vi "MC_10_19a_JW5.vi"() -> ()   [LabVIEW 2011]
uses:
  <vilib>/Utility/file.llb/Read From Spreadsheet File (string).vi
  <vilib>/Utility/inputDevices.llb/keyboardAcquire.vi
  <vilib>/Utility/file.llb/Write To Spreadsheet File (DBL).vi
  <vilib>/Utility/file.llb/Write To Spreadsheet File (string).vi
  <vilib>/regexp/Match Regular Expression.xnode
panel:
  out "Current \nRecord":string[](array[string])
  out "Transformer \nHeaders":string[](array[string])
  out "Current Device ID":string
  out "Column":string
  out "Row":string
  out "Date Recorded":string="Date Recorded"
  out "Concentration Recorded":string
  out "Solvent Recorded":string
  out "Method Recorded":string
  in  "?":T1(tab)
  out "Material Recorded":string
  in  "Treatment Concentration (mM):":dbl=30.0
  in  "Surface Treatment:":string
  in  "# Drops:":dbl=inf
  in  "Solution Temp (C):":dbl=55.0
  in  "Relative Humidity (%):":dbl=nan
  in  "Room Temp (F):":dbl=nan
  in  "Time (s):":dbl=80.0
  out "Accel (RPM/s):":dbl
  in  "RPM:":dbl=1000.0
  in  "Wait Time (s):":dbl=10.0
  in  "Sample #:":dbl=1.0
  in  "Fabricator:":string="Jeremy"
  in  "Data File":path
  out "Data Folder":path
  in  "Image Folder":path
  out "Image File":path
  in  "Ramp (s):":dbl=3.0
  out "Mobility":dbl format="%#_4e"
  out "Length":dbl
  out "Width":dbl
  out "Dielectric (d)":dbl
  out "XY Graph":cluster{dbl[], dbl[]}[](graph)
  in  "NumPts":dbl=5.0
  in  "Cancel Button":bool
  in  "Next Button":bool
  in  "Previous Button":bool
  in  "Up Button":bool
  in  "Down Button":bool
  out "Data Name":string
  in  "Save Changes?":bool
  in  "New Dielectric":dbl
  in  "New Length":dbl
  in  "New Width":dbl
  out "New Mobility":dbl format="%#_4e"
  in  "Slide":dbl(slide) step=1.0 scale=-14.3..84.0 scale format="%#_1p"
  in  "Blank Button":bool
  in  "Zoom":i16(slide)=-3 scale=-5.0..5.0
  out "Image Out 2":T2(plugin-control)
  out "Image Out":T2(plugin-control)
  in  "Magnification":u16(ring) items=["5x", "10x", "20x", "50x", "80x"]
  out "Total Width":dbl
  out "Distances":dbl[](array[numeric])
  in  "Undo Button":bool
  in  "Remove Button":bool
  out "Recorded Mobility":dbl format="%#_4e"
  out "Index 3":string
  out "Image Name":string
  in  "Export":bool
  out "Threshold V":dbl
  out "New Vt":dbl
  in  "Manual":bool
  out "XY Graph 2":cluster{dbl[], dbl[]}[](graph)
  in  "Next Button 2":bool
  in  "Previous Button 2":bool
  in  "Slide 2":dbl(slide) step=1.0 scale=-1.0..82.0 scale format="%#_1p"
  out "S.T.S.":dbl
  out "New S.T.S.":dbl
  in  "NumPts 2":dbl=5.0
  out "Vt recorded":dbl
  out "STS recorded":dbl
  out "On/Off":dbl format="%#_3e"
  in  "Save Changes? 2":bool
  in  "Save Changes? 3":bool
  out "String":string
  in  "No Image":path=path "C:/Program Files/Mega Awesome/Image Not Found.png"
  in  "Project":path=path "C:/Program Files/Mega Awesome/DeviceData.opj"
  out "Index 2":dbl
  out "Array 8":dbl[](array[numeric])
  out "Array 7":dbl[](array[numeric])
  out "ROI Descriptor out":T3 {"Contours"."Type" items=["No Selection", "Point", "Line", "Rectangle", "Oval", "Polygon", "Freehand Region", "Annulus", "Unused2", "Unused3", "Broken Line", "Freehand Line", "Rotated Rectangle"]}
  out "ROI Descriptor":T3 {"Contours"."Type" items=["No Selection", "Point", "Line", "Rectangle", "Oval", "Polygon", "Freehand Region", "Annulus", "Unused2", "Unused3", "Broken Line", "Freehand Line", "Rotated Rectangle"]}
  out "Numeric 3":dbl
  out "Array 6":dbl[][](array[numeric])
  out "Cluster":T4
  out "Array 5":dbl[](array[numeric])
  out "Array 4":dbl[](array[numeric])
  out "Array 3":dbl[](array[numeric])
  out "Numeric 2":dbl
  out "Numeric":dbl
  out "Array 2":dbl[](array[numeric])
  out "Array":dbl[](array[numeric])
  out "Index":dbl
  out "Table Control 2":string[][](table)
  out "Table Control":string[][](table)
  in  "Row Start":dbl=20.0
  # "Data Locations"
  # "Data Location"
  # "Image Location"
  # "Sample Properties"
  # "Recorded"
  # "Calculated"
  # "Re-Calculated"
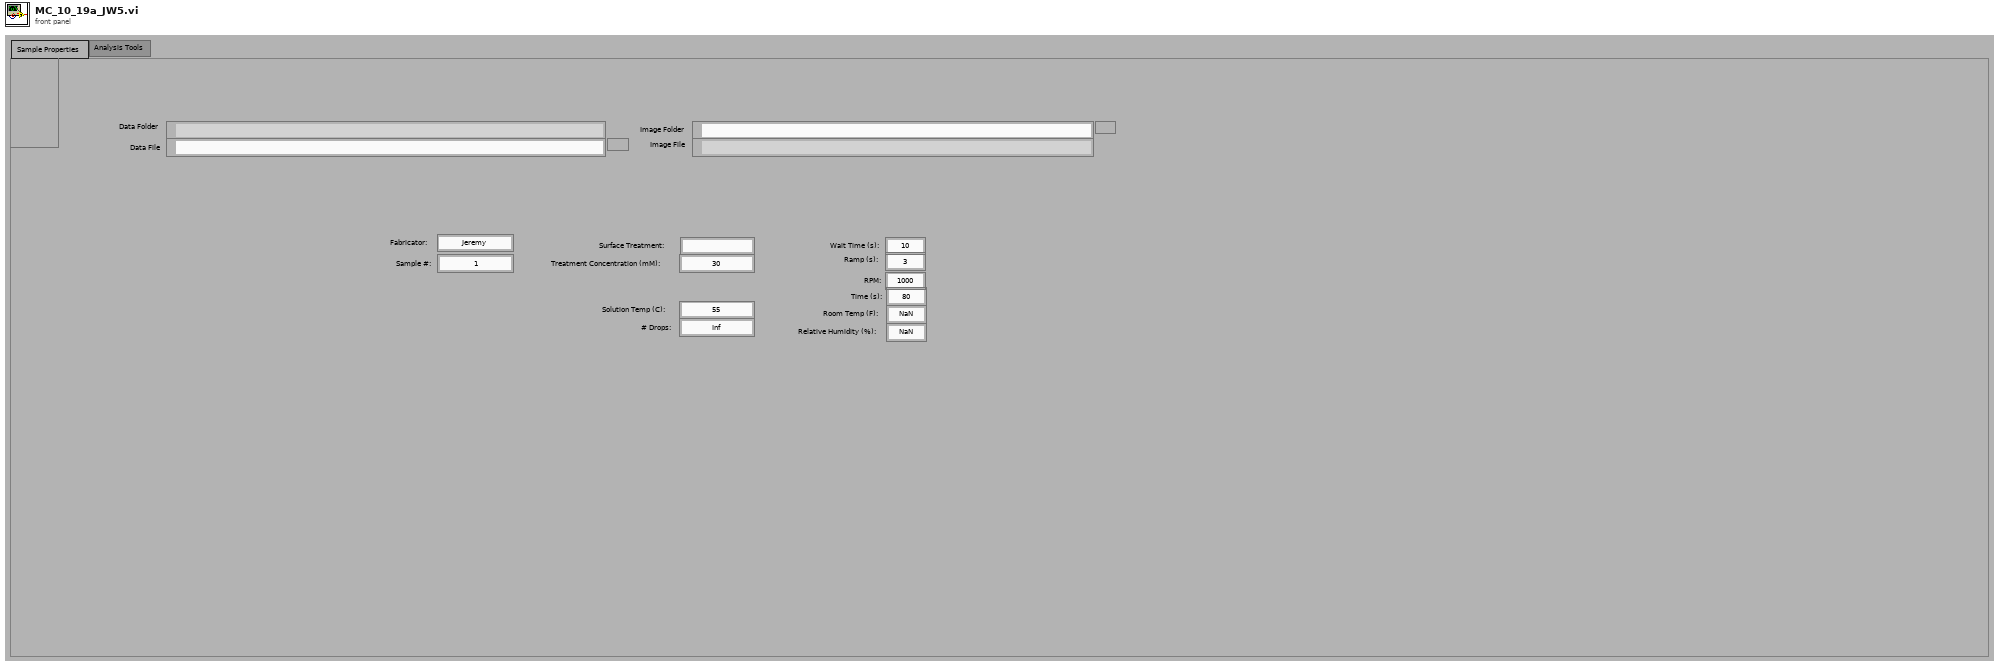
[diagram p1: front panel]
types:
  T1 = enum32{"Sample Properties", "Analysis Tools", "Current Database"}
  T2 = typedef "IMAQ Image.ctl" = refnum<image>
  T3 = typedef "ROI Descriptor" = cluster{"Global Rectangle":i32[], "Contours":cluster{"ID":enum32{"External", "Internal"}, "Type":u32, "Coordinates":i32[]}[]}
  T4 = cluster{"Numeric":dbl, "Numeric 2":dbl, "Numeric 3":dbl, "Numeric 4":dbl}
  T5 = cluster{"[0]":cluster{dbl[], dbl[]}, "[1]":cluster{dbl[], dbl[]}, "[2]":cluster{dbl[], dbl[]}, "[3]":cluster{dbl[], dbl[]}, "[4]":cluster{dbl[], dbl[]}, "[5]":cluster{dbl[], dbl[]}, "[6]":cluster{dbl[], dbl[]}, "[7]":cluster{dbl[], dbl[]}, "[8]":cluster{dbl[], dbl[]}}
  T6 = cluster{"Vt":dbl, "STS":dbl, "On/Off":dbl, "Deposition":string, "Solvent":string, "Concentration":string, "Material":string}
  T7 = cluster{"Global Rectangle":i32[], "Contours":cluster{"Contour Type":u32, "ROI Type":u32, "Points":i32[]}[]}
  T8 = typedef "LVBoundsTypeDef.ctl" = cluster{"Width":u32, "Height":u32}
  T9 = cluster{"Contour Type":u32, "ROI Type":u32, "Points":i32[]}[]
  T10 = enum16{"0", "1", "2", "3", "4", "5", "6", "7", "8", "9", "A", "B", "C", "D", "E", "F", "G", "H", "I", "J", "K", "L", "M", "N", "O", "P", "Q", "R", "S", "T", "U", "V", "W", "X", "Y", "Z", "F1", "F2", "F3", "F4", "F5", "F6", "F7", "F8", "F9", "F10", "F11", "F12", "F13", "F14", "F15", "ADD", "BACK", "BACKSLASH", "CAPITAL", "COMMA", "DECIMAL", "DELETE", "DIVIDE", "DOWN", "END", "EQUALS", "ESCAPE", "GRAVE (`)", "HOME", "INSERT", "LBRACKET", "LCONTROL", "LEFT", "L ALT", "LSHIFT", "LWIN", "MINUS", "MULTIPLY", "NEXT", "NUMLOCK", "NUMPAD_0", "NUMPAD_1", "NUMPAD_2", "NUMPAD_3", "NUMPAD_4", "NUMPAD_5", "NUMPAD_6", "NUMPAD_7", "NUMPAD_8", "NUMPAD_9", "PAUSE", "PERIOD", "PRIOR (PG UP)", "RBRACKET", "RCONTROL", "RETURN", "RIGHT", "R ALT", "RSHIFT", "RWIN", "SCROLL", "SEMICOLON", "SLASH", "SPACE", "SUBTRACT", "TAB", "UP", "ENTER (num pad)", "' (quote)"}[]
  T11 = cluster{i32[], cluster{"Contour Type":u32, "ROI Type":u32, "Points":i32[]}[]}
  T12 = enum16{"0", "1", "2", "3", "4", "5", "6", "7", "8", "9", "A", "B", "C", "D", "E", "F", "G", "H", "I", "J", "K", "L", "M", "N", "O", "P", "Q", "R", "S", "T", "U", "V", "W", "X", "Y", "Z", "F1", "F2", "F3", "F4", "F5", "F6", "F7", "F8", "F9", "F10", "F11", "F12", "F13", "F14", "F15", "ADD", "BACK", "BACKSLASH", "CAPITAL", "COMMA", "DECIMAL", "DELETE", "DIVIDE", "DOWN", "END", "EQUALS", "ESCAPE", "GRAVE (`)", "HOME", "INSERT", "LBRACKET", "LCONTROL", "LEFT", "L ALT", "LSHIFT", "LWIN", "MINUS", "MULTIPLY", "NEXT", "NUMLOCK", "NUMPAD_0", "NUMPAD_1", "NUMPAD_2", "NUMPAD_3", "NUMPAD_4", "NUMPAD_5", "NUMPAD_6", "NUMPAD_7", "NUMPAD_8", "NUMPAD_9", "PAUSE", "PERIOD", "PRIOR (PG UP)", "RBRACKET", "RCONTROL", "RETURN", "RIGHT", "R ALT", "RSHIFT", "RWIN", "SCROLL", "SEMICOLON", "SLASH", "SPACE", "SUBTRACT", "TAB", "UP", "ENTER (num pad)", "' (quote)"}
  T13 = cluster{string, sgl, bool, bool, bool, bool, bool, bool, i32}
  T14 = cluster{i32, cluster{string, sgl, bool, bool, bool, bool, bool, bool, i32}, i32, i32}
  T15 = cluster{"Contour Type":u32, "ROI Type":u32, "Points":i32[]}
  T16 = cluster{"Points[0]":i32, "Points[1]":i32, "Points[2]":i32, "Points[3]":i32, "Points[4]":i32, "Points[5]":i32, "Points[6]":i32, "Points[7]":i32, "Points[8]":i32}
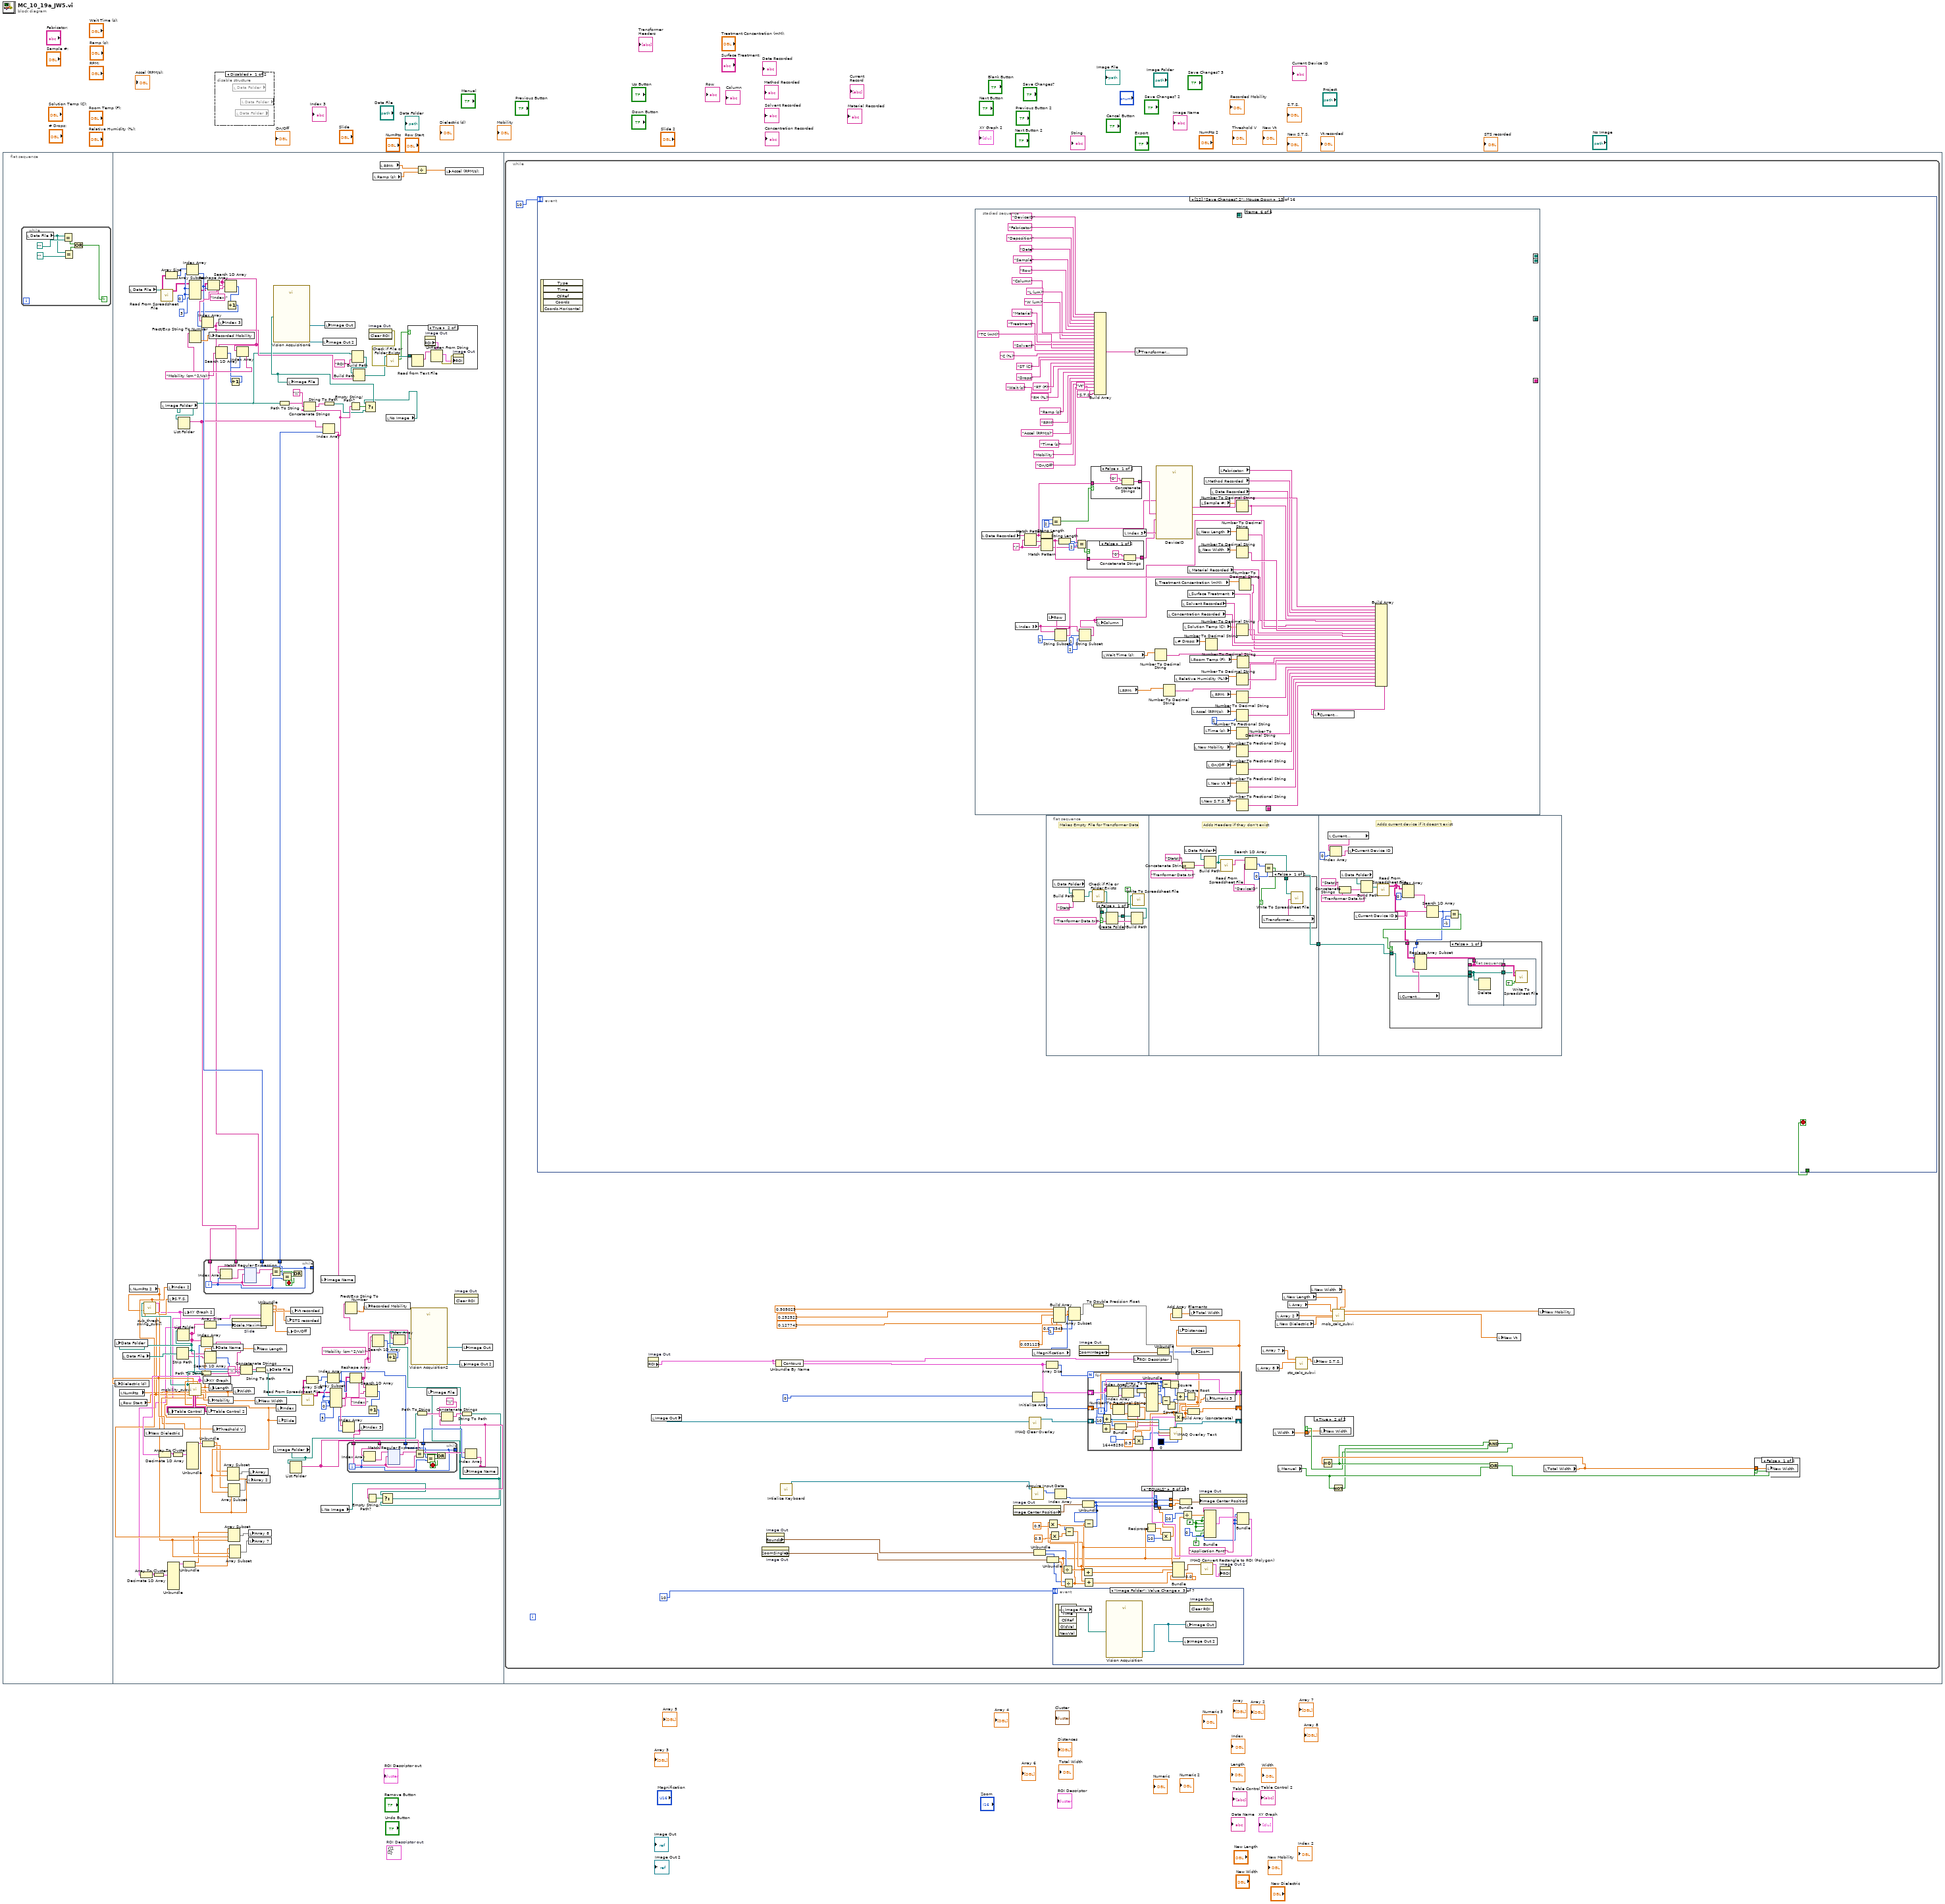
[diagram p0: block diagram]
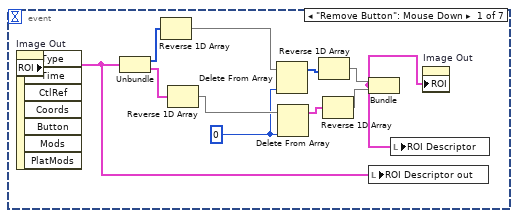
[diagram p5: hidden frame]
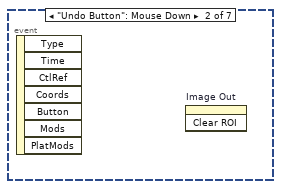
[diagram p6: hidden frame]
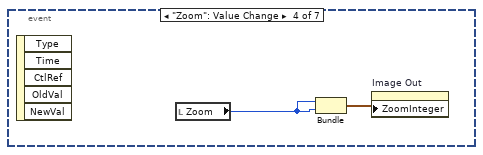
[diagram p7: hidden frame]
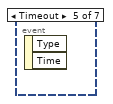
[diagram p8: hidden frame]
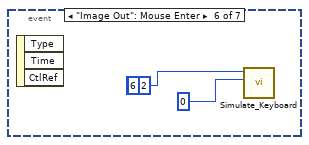
[diagram p9: hidden frame]
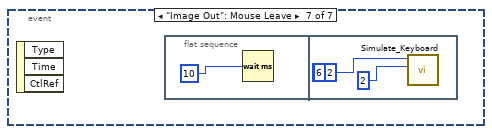
[diagram p10: hidden frame]
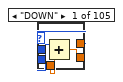
[diagram p11: hidden frame]
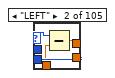
[diagram p12: hidden frame]
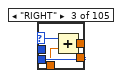
[diagram p13: hidden frame]
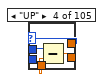
[diagram p14: hidden frame]
diagram:
  (unwired) T3 {"Global Rectangle"=[], "Contours"=[]}  # ROI Descriptor out
  n1 = flat-sequence {
    frame #0 {
      n2 = while {
        stop <- w1 continue-if-true
        n3 = local read "Data File"() -> (w3:path)
        n4 = Equal?(x=w3, y=path "") -> (x = y?=w5:bool)
        n5 = Equal?(x=w3, y=path "") -> (x = y?=w4:bool)
        n6 = Or(x=w5, y=w4) -> (x .or. y?=w1:bool)
      }
    }
    frame #1 {
      w70 = 0
      w100 = 0
      n7 = local read "NumPts"() -> (w45:dbl)
      n8 = local read "Row Start"() -> (w44:dbl)
      n9 = local read "Data File"() -> (w74:path)
      n10 = local read "Data File"() -> (w95:path)
      n11 = local read "NumPts 2"() -> (w39:dbl)
      n12 = call-poly <vilib>:"Read From Spreadsheet File.vi"("file path (dialog if empty)"=w95) -> ("all rows"=w98:string[][])  [unwired: 6 in, 4 out]
      n13 = local read "Image Folder"() -> (w10:path)
      n14 = Array Size(array=w98) -> (size(s)=w99:i32[])
      n15 = Strip Path(path=w74) -> (stripped path=w75:path, name=w56:string)
      n16 = local write "Data Folder"(w75) -> ()
      n17 = List Folder(path=w75) -> (filenames=w64:string[])  [unwired: 3 in, 3 out]
      n18 = List Folder(path=w10) -> (filenames=w104:string[])  [unwired: 3 in, 3 out]
      n19 = Index Array(array=w99, index=w100) -> (element=w106:i32)
      n20 = Array Subset(array=w98, index (row)=w100, index (col)=w100, length (col)=3) -> (w97:string[][])  [unwired: 1 in]
      n21 = Path To String(path=w75) -> (string=w55:string)
      n22 = Array Size(array=w64) -> (size(s)=w65:i32)
      n23 = Search 1D Array(1D array=w64, element=w56) -> (index of element=w63:i32)  [unwired: 1 in]
      n24 = Index Array(array=w64, index=w63) -> (element=w62:string)
      n25 = Reshape Array(w97, w106) -> (w116:string[])
      n26 = local write "Data Name"(w62) -> ()
      n27 = Search 1D Array(1D array=w116, element="Mobility (cm^2/Vs):") -> (index of element=w111:i32)  [unwired: 1 in]
      n28 = Search 1D Array(1D array=w116, element="Index:") -> (index of element=w103:i32)  [unwired: 1 in]
      n29 = Increment(x=w103) -> (x+1=w102:i32)
      n30 = Index Array(array=w116, index=w102) -> (element=w11:string)
      n31 = while {
        tunnel: w104 -> [w249]
        tunnel: w11 -> [w247]
        tunnel: [w246] -> _
        tunnel: [w246] -> w105
        tunnel: w106 -> [w245]
        i -> [w246]
        stop <- w242 stop-if-true
        n32 = Index Array(array=w249, index=w246) -> (element=w250:string)
        n33 = xnode "Match Regular Expression"("input string"=w250, "regular expression"=w247) -> ("whole match"=w248:string)  [unwired: 4 in, 4 out]
        n34 = Equal?(x=w248, y=w247) -> (x = y?=w244:bool)
        n35 = Equal?(x=w245, y=w246) -> (x = y?=w243:bool)
        n36 = Or(x=w244, y=w243) -> (x .or. y?=w242:bool)
      }
      n37 = local write "Index 3"(w11) -> ()
      n38 = Increment(x=w111) -> (x+1=w112:i32)
      n39 = property on="Slide" class="Slide (strict)"("Scale.Maximum"=w65) -> ()  [unwired: 2 in, 2 out]
      n40 = Index Array(array=w116, index=w112) -> (element=w114:string)
      n41 = Fract/Exp String To Number(string=w114) -> (number=w115:dbl)  [unwired: 3 in, 1 out]
      n42 = local write "Recorded Mobility"(w115) -> ()
      n43 = Concatenate Strings(w55, "\\", w62) -> (w57:string)
      n44 = String To Path(string=w57) -> (path=w46:path)
      n45 = call "sub_thresh_swing_subvi.vi"("Path"=w46, "NumPts"=w39, "Row Start"=w44) -> ("Index"=w40:dbl, "XY Graph"=w35:cluster{dbl[], dbl[]}[], "Sub Threshold Swing"=w47:dbl)  [unwired: 8 in, 2 out]
      n46 = Decimate 1D Array(w35) -> (w36:cluster{dbl[], dbl[]}[])  [unwired: 1 out]
      n47 = Array To Cluster(array=w36) -> (cluster=w38:T5)
      n48 = local write "Index 2"(w40) -> ()
      n49 = Unbundle(w38) -> ("[0]"=w37:cluster{dbl[], dbl[]})  [unwired: 8 out]
      n50 = local write "S.T.S."(w47) -> ()
      n51 = local write "XY Graph 2"(w35) -> ()
      n52 = Unbundle(w37) -> (w33:dbl[], w32:dbl[])
      n53 = call "mobility_subvi.vi"("Path"=w46, "NumPts"=w45, "Row Start"=w44) -> ("Dielectric (d)"=w51:dbl, "Index"=w52:dbl, "XY Graph"=w94:cluster{dbl[], dbl[]}[], "Length"=w50:dbl, "Vt"=w48:dbl, "Width"=w49:dbl, "Table Control"=w59:string[][], "Table Control 2"=w60:string[][], "Recorded"=w29:T6, "Mobility"=w61:dbl)  [unwired: 2 in, 1 out]
      n54 = local write "Dielectric (d)"(w51) -> ()
      n55 = local write "New Dielectric"(w51) -> ()
      n56 = Decimate 1D Array(w94) -> (w93:cluster{dbl[], dbl[]}[])  [unwired: 1 out]
      n57 = local write "Table Control"(w59) -> ()
      n58 = Array To Cluster(array=w93) -> (cluster=w91:T5)
      n59 = Unbundle(w91) -> ("[0]"=w92:cluster{dbl[], dbl[]})  [unwired: 8 out]
      n60 = Unbundle(w92) -> (w34:dbl[], w41:dbl[])
      n61 = local write "XY Graph"(w94) -> ()
      n62 = local write "Table Control 2"(w60) -> ()
      n63 = local write "Mobility"(w61) -> ()
      n64 = local write "Length"(w50) -> ()
      n65 = local write "Threshold V"(w48) -> ()
      n66 = Array Subset(array=w34, index=w52, length=w45) -> (w53:dbl[])
      n67 = Array Subset(array=w41, index=w52, length=w45) -> (w54:dbl[])
      n68 = Array Subset(array=w33, index=w40, length=w39) -> (w43:dbl[])
      n69 = Array Subset(array=w32, index=w40, length=w39) -> (w42:dbl[])
      n70 = local write "Width"(w49) -> ()
      n71 = local write "Array 2"(w54) -> ()
      n72 = local write "Array 8"(w43) -> ()
      n73 = local write "Array 7"(w42) -> ()
      n74 = local write "Array"(w53) -> ()
      n75 = local write "New Length"(w50) -> ()
      n76 = local write "New Width"(w49) -> ()
      n77 = Unbundle(w29) -> ("Vt"=w31:dbl, "STS"=w30:dbl, "On/Off"=w28:dbl)  [unwired: 4 out]
      n78 = local write "Data File"(w46) -> ()
      n79 = local read "Image Folder"() -> (w81:path)
      n80 = local write "Index"(w52) -> ()
      n81 = local write "Slide"(w52) -> ()
      n82 = Path To String(path=w10) -> (string=w108:string)
      n83 = local write "STS recorded"(w30) -> ()
      n84 = local write "On/Off"(w28) -> ()
      n85 = List Folder(path=w81) -> (filenames=w77:string[])  [unwired: 3 in, 3 out]
      n86 = local write "Vt recorded"(w31) -> ()
      n87 = call-poly <vilib>:"Read From Spreadsheet File.vi"("file path (dialog if empty)"=w46) -> ("all rows"=w68:string[][])  [unwired: 6 in, 4 out]
      n88 = Array Size(array=w68) -> (size(s)=w69:i32[])
      n89 = local read "No Image"() -> (w19:path)
      n90 = Index Array(array=w104, index=w105) -> (element=w27:string)
      n91 = Concatenate Strings(w108, "\\", w27) -> (w109:string)
      n92 = local write "Image Name"(w27) -> ()
      n93 = String To Path(string=w109) -> (path=w25:path)
      n94 = Index Array(array=w69, index=w70) -> (element=w80:i32)
      n95 = Array Subset(array=w68, index (row)=w70, index (col)=w70, length (col)=3) -> (w67:string[][])  [unwired: 1 in]
      n96 = Empty String/Path?(string/path=w27) -> (empty?=w26:bool)
      n97 = Reshape Array(w67, w80) -> (w90:string[])
      n98 = Build Path(base path=w10, name or relative path="ROI") -> (appended path=w13:path)
      n99 = Build Path(base path=w13, name or relative path=w11) -> (appended path=w12:path)
      n100 = Search 1D Array(1D array=w90, element="Index:") -> (index of element=w73:i32)  [unwired: 1 in]
      n101 = Increment(x=w73) -> (x+1=w72:i32)
      n102 = Index Array(array=w90, index=w72) -> (element=w78:string)
      n103 = while {
        tunnel: w77 -> [w129]
        tunnel: w78 -> [w127]
        tunnel: [w126] -> _
        tunnel: [w126] -> w79
        tunnel: w80 -> [w125]
        i -> [w126]
        stop <- w122 stop-if-true
        n104 = Index Array(array=w129, index=w126) -> (element=w130:string)
        n105 = xnode "Match Regular Expression"("input string"=w130, "regular expression"=w127) -> ("whole match"=w128:string)  [unwired: 4 in, 4 out]
        n106 = Equal?(x=w128, y=w127) -> (x = y?=w124:bool)
        n107 = Equal?(x=w125, y=w126) -> (x = y?=w123:bool)
        n108 = Or(x=w124, y=w123) -> (x .or. y?=w122:bool)
      }
      n109 = local write "Index 3"(w78) -> ()
      n110 = invoke on="Image Out" class="ImageControl" method="Clear ROI"() -> (error out=w17:errorcluster)  [unwired: 3 in, 2 out]
      n111 = Search 1D Array(1D array=w90, element="Mobility (cm^2/Vs):") -> (index of element=w85:i32)  [unwired: 1 in]
      n112 = local read "Ramp (s):"() -> (w8:dbl)
      n113 = local read "RPM:"() -> (w7:dbl)
      n114 = local read "No Image"() -> (w18:path)
      n115 = Select(t=w18, s=w26, f=w25) -> (s? t:f=w24:path)
      n116 = call "Vision Acquisition6"("Image Path"=w24) -> ("Image Out"=w107:T2)  [unwired: 25 in, 1 out]
      n117 = local write "Image File"(w24) -> ()
      n118 = local write "Image Out 2"(w107) -> ()
      n119 = local write "Image Out"(w107) -> ()
      n120 = Increment(x=w85) -> (x+1=w86:i32)
      n121 = call <vilib>:"Check if File or Folder Exists.vi"("error in (no error)"=w17, "path"=w12) -> ("file or folder exists?"=w15:bool, "dup path"=w16:path)  [unwired: 7 in, 1 out]
      n122 = Index Array(array=w90, index=w86) -> (element=w88:string)
      n123 = Fract/Exp String To Number(string=w88) -> (number=w89:dbl)  [unwired: 3 in, 1 out]
      n124 = local write "Recorded Mobility"(w89) -> ()
      n125 = case shown="True" w15 {
        tunnel: w16 -> [_ w117]
        frame False {
        }
        frame True {
          n126 = Read from Text File(file (use dialog)=w117) -> (text=w121:string)  [unwired: 3 in, 3 out]
          n127 = property on="Image Out" class="ImageControl"() -> ("ROI"=w118:T7)  [unwired: 2 in, 2 out]
          n128 = Unflatten From String(type=w118, binary string=w121) -> (value=w119:T7, error out=w120:errorcluster)  [unwired: 3 in, 1 out]
          n129 = property on="Image Out" class="ImageControl"(error in=w120, "ROI"=w119) -> ()  [unwired: 1 in, 2 out]
        }
      }
      n130 = Divide(x=w7, y=w8) -> (x/y=w9:dbl)
      n131 = Path To String(path=w81) -> (string=w82:string)
      n132 = local write "Accel (RPM/s):"(w9) -> ()
      n133 = invoke on="Image Out" class="ImageControl" method="Clear ROI"() -> ()  [unwired: 3 in, 3 out]
      n134 = Index Array(array=w77, index=w79) -> (element=w22:string)
      n135 = Empty String/Path?(string/path=w22) -> (empty?=w23:bool)
      n136 = Concatenate Strings(w82, "\\", w22) -> (w83:string)
      n137 = String To Path(string=w83) -> (path=w21:path)
      n138 = Select(t=w19, s=w23, f=w21) -> (s? t:f=w20:path)
      n139 = call "Vision Acquisition2"("Image Path"=w20) -> ("Image Out"=w76:T2)  [unwired: 25 in, 1 out]
      n140 = local write "Image File"(w20) -> ()
      n141 = local write "Image Out 2"(w76) -> ()
      n142 = local write "Image Out"(w76) -> ()
      n143 = local write "Image Name"(w22) -> ()
    }
    frame #2 {
      n144 = while {
        stop <- w441 stop-if-true
        w391 = FALSE
        w389 = 0
        n145 = event shown="[12] \"Save Changes? 2\": Mouse Down" {
          selector: _ -> [_ _ _ _ _ _ _ _ _ _ _ _ _ _ _ _]
          dyn-events: _ -> [_ _ _ _ _ _ _ _ _ _ _ _ _ _ _ _]
          timeout: 10 -> [_ _ _ _ _ _ _ _ _ _ _ _ _ _ _ _]
          tunnel: [_ _ _ _ _ _ _ _ _ _ _ _ _ TRUE _ TRUE] -> w441
          event Timeout {
            n146 = event-data() -> ()  [unwired: 1 in, 2 out]
          }
          event "Down Button": Mouse Down {
            w789 = 0
            n147 = event-data() -> ()  [unwired: 1 in, 7 out]
            n148 = local read "NumPts 2"() -> (w750:dbl)
            n149 = local read "NumPts"() -> (w757:dbl)
            n150 = local read "Row Start"() -> (w756:dbl)
            n151 = local read "Data File"() -> (w794:path)
            n152 = property on="Image Out" class="ImageControl"() -> (error out=w719:errorcluster, "Image Center Position"=w723:cluster{"X":u32, "Y":u32})  [unwired: 2 in, 1 out]
            n153 = Unbundle(w723) -> ("X"=w721:u32)  [unwired: 1 out]
            n154 = Strip Path(path=w794) -> (stripped path=w785:path, name=w807:string)
            n155 = local write "Data Folder"(w785) -> ()
            n156 = List Folder(path=w785) -> (filenames=w800:string[], error out=w728:errorcluster)  [unwired: 3 in, 2 out]
            n157 = Array Size(array=w800) -> (size(s)=w795:i32)
            n158 = Bundle("X"=w721, 0) -> (w722:cluster{"X":u32, i32})  [unwired: 1 in]
            n159 = Path To String(path=w785) -> (string=w808:string)
            n160 = Search 1D Array(1D array=w800, element=w807) -> (index of element=w797:i32)  [unwired: 1 in]
            n161 = property on="Image Out" class="ImageControl"(error in=w719, "Image Center Position"=w722) -> ()  [unwired: 1 in, 2 out]
            n162 = Decrement(x=w795) -> (x-1=w798:i32)
            n163 = Equal?(x=w797, y=w798) -> (x = y?=w799:bool)
            n164 = case shown="False" w799 {
              tunnel: w797 -> [w935 _]
              tunnel: [w934 0] -> w796
              frame False {
                n165 = Increment(x=w935) -> (x+1=w934:i32)
              }
              frame True {
              }
            }
            n166 = Index Array(array=w800, index=w796) -> (element=w801:string)
            n167 = local write "Data Name"(w801) -> ()
            n168 = Concatenate Strings(w808, "\\", w801) -> (w806:string)
            n169 = String To Path(string=w806) -> (path=w758:path)
            n170 = call "sub_thresh_swing_subvi.vi"("Path"=w758, "NumPts"=w750, "Row Start"=w756) -> ("Index"=w751:dbl, "XY Graph"=w746:cluster{dbl[], dbl[]}[], "Sub Threshold Swing"=w759:dbl)  [unwired: 8 in, 2 out]
            n171 = Decimate 1D Array(w746) -> (w749:cluster{dbl[], dbl[]}[])  [unwired: 1 out]
            n172 = Array To Cluster(array=w749) -> (cluster=w747:T5)
            n173 = Unbundle(w747) -> ("[0]"=w748:cluster{dbl[], dbl[]})  [unwired: 8 out]
            n174 = Unbundle(w748) -> (w745:dbl[], w744:dbl[])
            n175 = local write "S.T.S."(w759) -> ()
            n176 = local write "XY Graph 2"(w746) -> ()
            n177 = local write "Index 2"(w751) -> ()
            n178 = call "mobility_subvi.vi"("Path"=w758, "NumPts"=w757, "Row Start"=w756) -> ("Dielectric (d)"=w761:dbl, "Date Created"=w718:string, "Index"=w766:dbl, "XY Graph"=w769:cluster{dbl[], dbl[]}[], "Length"=w760:dbl, "Vt"=w762:dbl, "Width"=w734:dbl, "Table Control"=w804:string[][], "Table Control 2"=w803:string[][], "Recorded"=w743:T6, "Mobility"=w802:dbl)  [unwired: 2 in]
            n179 = local write "Dielectric (d)"(w761) -> ()
            n180 = local write "Threshold V"(w762) -> ()
            n181 = local write "New Dielectric"(w761) -> ()
            n182 = Decimate 1D Array(w769) -> (w770:cluster{dbl[], dbl[]}[])  [unwired: 1 out]
            n183 = Array To Cluster(array=w770) -> (cluster=w772:T5)
            n184 = local write "Table Control"(w804) -> ()
            n185 = Unbundle(w772) -> ("[0]"=w771:cluster{dbl[], dbl[]})  [unwired: 8 out]
            n186 = Unbundle(w771) -> (w753:dbl[], w752:dbl[])
            n187 = local write "XY Graph"(w769) -> ()
            n188 = local write "Table Control 2"(w803) -> ()
            n189 = local write "Mobility"(w802) -> ()
            n190 = Array Subset(array=w753, index=w766, length=w757) -> (w768:dbl[])
            n191 = Array Subset(array=w752, index=w766, length=w757) -> (w767:dbl[])
            n192 = Unbundle(w743) -> ("Vt"=w742:dbl, "STS"=w741:dbl, "On/Off"=w740:dbl, "Deposition"=w717:string, "Solvent"=w716:string, "Concentration"=w715:string, "Material"=w714:string)
            n193 = local write "On/Off"(w740) -> ()
            n194 = local write "Width"(w734) -> ()
            n195 = local write "Length"(w760) -> ()
            n196 = local write "Array 2"(w767) -> ()
            n197 = local write "Array"(w768) -> ()
            n198 = local write "Slide"(w766) -> ()
            n199 = local write "Index"(w766) -> ()
            n200 = local write "STS recorded"(w741) -> ()
            n201 = local write "Date Recorded"(w718) -> ()
            n202 = local write "Solvent Recorded"(w716) -> ()
            n203 = local write "Concentration Recorded"(w715) -> ()
            n204 = local write "Method Recorded"(w717) -> ()
            n205 = local write "Vt recorded"(w742) -> ()
            n206 = Array Subset(array=w745, index=w751, length=w750) -> (w755:dbl[])
            n207 = Array Subset(array=w744, index=w751, length=w750) -> (w754:dbl[])
            n208 = local write "Material Recorded"(w714) -> ()
            n209 = local write "New Width"(w734) -> ()
            n210 = local write "Data File"(w758) -> ()
            n211 = local write "New Length"(w760) -> ()
            n212 = local write "Array 8"(w755) -> ()
            n213 = local write "Array 7"(w754) -> ()
            n214 = call-poly <vilib>:"Read From Spreadsheet File.vi"("file path (dialog if empty)"=w758) -> ("all rows"=w791:string[][])  [unwired: 6 in, 4 out]
            n215 = local read "Image Folder"() -> (w725:path)
            n216 = Array Size(array=w791) -> (size(s)=w790:i32[])
            n217 = List Folder(path=w725, error in=w728) -> (filenames=w784:string[], error out=w729:errorcluster)  [unwired: 2 in, 2 out]
            n218 = Index Array(array=w790, index=w789) -> (element=w764:i32)
            n219 = Subtract(x=w764, y=20) -> (x-y=w763:i32)
            n220 = property on="Slide" class="Slide (strict)"("Scale.Maximum"=w763) -> ()  [unwired: 2 in, 2 out]
            n221 = Array Subset(array=w791, index (row)=w789, index (col)=w789, length (col)=3) -> (w792:string[][])  [unwired: 1 in]
            n222 = Reshape Array(w792, w764) -> (w773:string[])
            n223 = local read "No Image"() -> (w735:path)
            n224 = Search 1D Array(1D array=w773, element="Mobility (cm^2/Vs):") -> (index of element=w778:i32)  [unwired: 1 in]
            n225 = Search 1D Array(1D array=w773, element="Index:") -> (index of element=w786:i32)  [unwired: 1 in]
            n226 = Increment(x=w786) -> (x+1=w787:i32)
            n227 = Index Array(array=w773, index=w787) -> (element=w727:string)
            n228 = while {
              tunnel: w784 -> [w821]
              tunnel: w727 -> [w819]
              tunnel: [w818] -> _
              tunnel: [w818] -> w783
              tunnel: w764 -> [w817]
              i -> [w818]
              stop <- w814 stop-if-true
              n229 = Index Array(array=w821, index=w818) -> (element=w822:string)
              n230 = xnode "Match Regular Expression"("input string"=w822, "regular expression"=w819) -> ("whole match"=w820:string)  [unwired: 4 in, 4 out]
              n231 = Equal?(x=w820, y=w819) -> (x = y?=w816:bool)
              n232 = Equal?(x=w817, y=w818) -> (x = y?=w815:bool)
              n233 = Or(x=w816, y=w815) -> (x .or. y?=w814:bool)
            }
            n234 = local write "Index 3"(w727) -> ()
            n235 = Increment(x=w778) -> (x+1=w777:i32)
            n236 = Build Path(base path=w725, name or relative path="ROI") -> (appended path=w724:path)
            n237 = Index Array(array=w773, index=w777) -> (element=w775:string)
            n238 = Fract/Exp String To Number(string=w775) -> (number=w774:dbl)  [unwired: 3 in, 1 out]
            n239 = local write "Recorded Mobility"(w774) -> ()
            n240 = Build Path(base path=w724, name or relative path=w727) -> (appended path=w733:path)
            n241 = Path To String(path=w725) -> (string=w781:string)
            n242 = invoke on="Image Out" class="ImageControl" method="Clear ROI"(error in=w729) -> (error out=w732:errorcluster)  [unwired: 2 in, 2 out]
            n243 = call <vilib>:"Check if File or Folder Exists.vi"("error in (no error)"=w732, "path"=w733) -> ("file or folder exists?"=w730:bool, "dup path"=w731:path)  [unwired: 7 in, 1 out]
            n244 = Index Array(array=w784, index=w783) -> (element=w738:string)
            n245 = Empty String/Path?(string/path=w738) -> (empty?=w739:bool)
            n246 = Concatenate Strings(w781, "\\", w738) -> (w780:string)
            n247 = String To Path(string=w780) -> (path=w737:path)
            n248 = Select(t=w735, s=w739, f=w737) -> (s? t:f=w736:path)
            n249 = call "Vision Acquisition4"("Image Path"=w736) -> ("Image Out"=w782:T2)  [unwired: 25 in, 1 out]
            n250 = local write "Image File"(w736) -> ()
            n251 = local write "Image Name"(w738) -> ()
            n252 = local write "Image Out 2"(w782) -> ()
            n253 = local write "Image Out"(w782) -> ()
            n254 = invoke on="Image Out" class="ImageControl" method="Clear ROI"() -> ()  [unwired: 3 in, 3 out]
            n255 = case shown="True" w730 {
              tunnel: w731 -> [_ w809]
              frame False {
              }
              frame True {
                n256 = Read from Text File(file (use dialog)=w809) -> (text=w813:string)  [unwired: 3 in, 3 out]
                n257 = property on="Image Out" class="ImageControl"() -> ("ROI"=w810:T7)  [unwired: 2 in, 2 out]
                n258 = Unflatten From String(type=w810, binary string=w813) -> (value=w811:T7, error out=w812:errorcluster)  [unwired: 3 in, 1 out]
                n259 = property on="Image Out" class="ImageControl"(error in=w812, "ROI"=w811) -> ()  [unwired: 1 in, 2 out]
              }
            }
          }
          event "Data File": Value Change {
            w1008 = 0
            n260 = event-data() -> ()  [unwired: 1 in, 5 out]
            n261 = local read "NumPts"() -> (w976:dbl)
            n262 = local read "Row Start"() -> (w975:dbl)
            n263 = local read "Data File"() -> (w1004:path)
            n264 = local read "NumPts 2"() -> (w969:dbl)
            n265 = property on="Image Out" class="ImageControl"() -> (error out=w937:errorcluster, "Image Center Position"=w941:cluster{"X":u32, "Y":u32})  [unwired: 2 in, 1 out]
            n266 = Strip Path(path=w1004) -> (stripped path=w1003:path, name=w1021:string)
            n267 = local write "Data Folder"(w1003) -> ()
            n268 = List Folder(path=w1003) -> (filenames=w1013:string[], error out=w947:errorcluster)  [unwired: 3 in, 2 out]
            n269 = Unbundle(w941) -> ("X"=w939:u32)  [unwired: 1 out]
            n270 = Path To String(path=w1003) -> (string=w1022:string)
            n271 = Search 1D Array(1D array=w1013, element=w1021) -> (index of element=w1014:i32)  [unwired: 1 in]
            n272 = Index Array(array=w1013, index=w1014) -> (element=w1015:string)
            n273 = Bundle("X"=w939, 0) -> (w940:cluster{"X":u32, i32})  [unwired: 1 in]
            n274 = local write "Data Name"(w1015) -> ()
            n275 = property on="Image Out" class="ImageControl"(error in=w937, "Image Center Position"=w940) -> ()  [unwired: 1 in, 2 out]
            n276 = Concatenate Strings(w1022, "\\", w1015) -> (w1020:string)
            n277 = String To Path(string=w1020) -> (path=w977:path)
            n278 = call "sub_thresh_swing_subvi.vi"("Path"=w977, "NumPts"=w969, "Row Start"=w975) -> ("Index"=w970:dbl, "XY Graph"=w965:cluster{dbl[], dbl[]}[], "Sub Threshold Swing"=w974:dbl)  [unwired: 8 in, 2 out]
            n279 = Decimate 1D Array(w965) -> (w968:cluster{dbl[], dbl[]}[])  [unwired: 1 out]
            n280 = Array To Cluster(array=w968) -> (cluster=w966:T5)
            n281 = Unbundle(w966) -> ("[0]"=w967:cluster{dbl[], dbl[]})  [unwired: 8 out]
            n282 = Unbundle(w967) -> (w963:dbl[], w962:dbl[])
            n283 = local write "Index 2"(w970) -> ()
            n284 = call "mobility_subvi.vi"("Path"=w977, "NumPts"=w976, "Row Start"=w975) -> ("Dielectric (d)"=w979:dbl, "Index"=w984:dbl, "XY Graph"=w987:cluster{dbl[], dbl[]}[], "Length"=w978:dbl, "Vt"=w980:dbl, "Width"=w952:dbl, "Table Control"=w1018:string[][], "Table Control 2"=w1017:string[][], "Recorded"=w959:T6, "Mobility"=w1016:dbl)  [unwired: 2 in, 1 out]
            n285 = local write "Dielectric (d)"(w979) -> ()
            n286 = local write "New Dielectric"(w979) -> ()
            n287 = Decimate 1D Array(w987) -> (w988:cluster{dbl[], dbl[]}[])  [unwired: 1 out]
            n288 = local write "Table Control"(w1018) -> ()
            n289 = Array To Cluster(array=w988) -> (cluster=w990:T5)
            n290 = Unbundle(w990) -> ("[0]"=w989:cluster{dbl[], dbl[]})  [unwired: 8 out]
            n291 = local write "Threshold V"(w980) -> ()
            n292 = local write "S.T.S."(w974) -> ()
            n293 = Unbundle(w989) -> (w964:dbl[], w971:dbl[])
            n294 = local write "XY Graph"(w987) -> ()
            n295 = local write "Table Control 2"(w1017) -> ()
            n296 = local write "Mobility"(w1016) -> ()
            n297 = local write "Length"(w978) -> ()
            n298 = local write "XY Graph 2"(w965) -> ()
            n299 = Unbundle(w959) -> ("Vt"=w961:dbl, "STS"=w960:dbl, "On/Off"=w958:dbl)  [unwired: 4 out]
            n300 = local write "On/Off"(w958) -> ()
            n301 = Array Subset(array=w963, index=w970, length=w969) -> (w973:dbl[])
            n302 = Array Subset(array=w962, index=w970, length=w969) -> (w972:dbl[])
            n303 = local write "Width"(w952) -> ()
            n304 = Array Subset(array=w964, index=w984, length=w976) -> (w986:dbl[])
            n305 = Array Subset(array=w971, index=w984, length=w976) -> (w985:dbl[])
            n306 = local write "Array 8"(w973) -> ()
            n307 = local write "Array 7"(w972) -> ()
            n308 = local write "STS recorded"(w960) -> ()
            n309 = local write "Vt recorded"(w961) -> ()
            n310 = local write "New Length"(w978) -> ()
            n311 = local write "New Width"(w952) -> ()
            n312 = local write "Array 2"(w985) -> ()
            n313 = local write "Array"(w986) -> ()
            n314 = local write "Data File"(w977) -> ()
            n315 = local read "Image Folder"() -> (w943:path)
            n316 = local write "Index"(w984) -> ()
            n317 = local write "Slide"(w984) -> ()
            n318 = List Folder(path=w943, error in=w947) -> (filenames=w1001:string[], error out=w946:errorcluster)  [unwired: 2 in, 2 out]
            n319 = call-poly <vilib>:"Read From Spreadsheet File.vi"("file path (dialog if empty)"=w977) -> ("all rows"=w1010:string[][])  [unwired: 6 in, 4 out]
            n320 = Array Size(array=w1010) -> (size(s)=w1009:i32[])
            n321 = Index Array(array=w1009, index=w1008) -> (element=w983:i32)
            n322 = Subtract(x=w983, y=20) -> (x-y=w981:i32)
            n323 = property on="Slide" class="Slide (strict)"("Scale.Maximum"=w981) -> ()  [unwired: 2 in, 2 out]
            n324 = Array Subset(array=w1010, index (row)=w1008, index (col)=w1008, length (col)=3) -> (w1011:string[][])  [unwired: 1 in]
            n325 = Reshape Array(w1011, w983) -> (w991:string[])
            n326 = Search 1D Array(1D array=w991, element="Index:") -> (index of element=w1005:i32)  [unwired: 1 in]
            n327 = Increment(x=w1005) -> (x+1=w1006:i32)
            n328 = Index Array(array=w991, index=w1006) -> (element=w945:string)
            n329 = while {
              tunnel: w1001 -> [w1035]
              tunnel: w945 -> [w1033]
              tunnel: [w1032] -> _
              tunnel: [w1032] -> w1000
              tunnel: w983 -> [w1031]
              i -> [w1032]
              stop <- w1028 stop-if-true
              n330 = Index Array(array=w1035, index=w1032) -> (element=w1036:string)
              n331 = xnode "Match Regular Expression"("input string"=w1036, "regular expression"=w1033) -> ("whole match"=w1034:string)  [unwired: 4 in, 4 out]
              n332 = Equal?(x=w1034, y=w1033) -> (x = y?=w1030:bool)
              n333 = Equal?(x=w1031, y=w1032) -> (x = y?=w1029:bool)
              n334 = Or(x=w1030, y=w1029) -> (x .or. y?=w1028:bool)
            }
            n335 = local write "Index 3"(w945) -> ()
            n336 = Search 1D Array(1D array=w991, element="Mobility (cm^2/Vs):") -> (index of element=w996:i32)  [unwired: 1 in]
            n337 = Increment(x=w996) -> (x+1=w995:i32)
            n338 = Index Array(array=w991, index=w995) -> (element=w993:string)
            n339 = Fract/Exp String To Number(string=w993) -> (number=w992:dbl)  [unwired: 3 in, 1 out]
            n340 = local write "Recorded Mobility"(w992) -> ()
            n341 = Build Path(base path=w943, name or relative path="ROI") -> (appended path=w942:path)
            n342 = Path To String(path=w943) -> (string=w999:string)
            n343 = local read "No Image"() -> (w953:path)
            n344 = Build Path(base path=w942, name or relative path=w945) -> (appended path=w951:path)
            n345 = invoke on="Image Out" class="ImageControl" method="Clear ROI"(error in=w946) -> (error out=w950:errorcluster)  [unwired: 2 in, 2 out]
            n346 = Index Array(array=w1001, index=w1000) -> (element=w956:string)
            n347 = Empty String/Path?(string/path=w956) -> (empty?=w957:bool)
            n348 = Concatenate Strings(w999, "\\", w956) -> (w998:string)
            n349 = String To Path(string=w998) -> (path=w955:path)
            n350 = Select(t=w953, s=w957, f=w955) -> (s? t:f=w954:path)
            n351 = call "Vision Acquisition3"("Image Path"=w954) -> ("Image Out"=w1002:T2)  [unwired: 25 in, 1 out]
            n352 = local write "Image File"(w954) -> ()
            n353 = local write "Image Out 2"(w1002) -> ()
            n354 = local write "Image Out"(w1002) -> ()
            n355 = local write "Image Name"(w956) -> ()
            n356 = call <vilib>:"Check if File or Folder Exists.vi"("error in (no error)"=w950, "path"=w951) -> ("file or folder exists?"=w948:bool, "dup path"=w949:path)  [unwired: 7 in, 1 out]
            n357 = invoke on="Image Out" class="ImageControl" method="Clear ROI"() -> ()  [unwired: 3 in, 3 out]
            n358 = case shown="True" w948 {
              tunnel: w949 -> [_ w1023]
              frame False {
              }
              frame True {
                n359 = Read from Text File(file (use dialog)=w1023) -> (text=w1027:string)  [unwired: 3 in, 3 out]
                n360 = property on="Image Out" class="ImageControl"() -> ("ROI"=w1024:T7)  [unwired: 2 in, 2 out]
                n361 = Unflatten From String(type=w1024, binary string=w1027) -> (value=w1025:T7, error out=w1026:errorcluster)  [unwired: 3 in, 1 out]
                n362 = property on="Image Out" class="ImageControl"(error in=w1026, "ROI"=w1025) -> ()  [unwired: 1 in, 2 out]
              }
            }
          }
          event "Up Button": Mouse Down {
            w1219 = 0
            n363 = event-data() -> ()  [unwired: 1 in, 5 out]
            n364 = local read "NumPts"() -> (w1190:dbl)
            n365 = local read "Row Start"() -> (w1189:dbl)
            n366 = local read "Data File"() -> (w1215:path)
            n367 = local read "NumPts 2"() -> (w1184:dbl)
            n368 = property on="Image Out" class="ImageControl"() -> (error out=w1148:errorcluster, "Image Center Position"=w1152:cluster{"X":u32, "Y":u32})  [unwired: 2 in, 1 out]
            n369 = Strip Path(path=w1215) -> (stripped path=w1214:path, name=w1235:string)
            n370 = local write "Data Folder"(w1214) -> ()
            n371 = List Folder(path=w1214) -> (filenames=w1225:string[], error out=w1158:errorcluster)  [unwired: 3 in, 2 out]
            n372 = Path To String(path=w1214) -> (string=w1236:string)
            n373 = Search 1D Array(1D array=w1225, element=w1235) -> (index of element=w1227:i32)  [unwired: 1 in]
            n374 = Equal To 0?(x=w1227) -> (x = 0?=w1228:bool)
            n375 = Unbundle(w1152) -> ("X"=w1150:u32)  [unwired: 1 out]
            n376 = Bundle("X"=w1150, 0) -> (w1151:cluster{"X":u32, i32})  [unwired: 1 in]
            n377 = property on="Image Out" class="ImageControl"(error in=w1148, "Image Center Position"=w1151) -> ()  [unwired: 1 in, 2 out]
            n378 = Array Size(array=w1225) -> (size(s)=w1224:i32)
            n379 = case shown="True" w1228 {
              tunnel: w1227 -> [w1363 _]
              tunnel: [w1362 w1364] -> w1226
              tunnel: w1224 -> [_ w1365]
              frame False {
                n380 = Decrement(x=w1363) -> (x-1=w1362:i32)
              }
              frame True {
                n381 = Decrement(x=w1365) -> (x-1=w1364:i32)
              }
            }
            n382 = Index Array(array=w1225, index=w1226) -> (element=w1229:string)
            n383 = local write "Data Name"(w1229) -> ()
            n384 = Concatenate Strings(w1236, "\\", w1229) -> (w1234:string)
            n385 = String To Path(string=w1234) -> (path=w1191:path)
            n386 = call "sub_thresh_swing_subvi.vi"("Path"=w1191, "NumPts"=w1184, "Row Start"=w1189) -> ("Index"=w1183:dbl, "XY Graph"=w1179:cluster{dbl[], dbl[]}[], "Sub Threshold Swing"=w1192:dbl)  [unwired: 8 in, 2 out]
            n387 = Decimate 1D Array(w1179) -> (w1182:cluster{dbl[], dbl[]}[])  [unwired: 1 out]
            n388 = Array To Cluster(array=w1182) -> (cluster=w1180:T5)
            n389 = Unbundle(w1180) -> ("[0]"=w1181:cluster{dbl[], dbl[]})  [unwired: 8 out]
            n390 = Unbundle(w1181) -> (w1178:dbl[], w1177:dbl[])
            n391 = Array Subset(array=w1178, index=w1183, length=w1184) -> (w1186:dbl[])
            n392 = Array Subset(array=w1177, index=w1183, length=w1184) -> (w1185:dbl[])
            n393 = local write "S.T.S."(w1192) -> ()
            n394 = local write "Array 8"(w1186) -> ()
            n395 = local write "Array 7"(w1185) -> ()
            n396 = call "mobility_subvi.vi"("Path"=w1191, "NumPts"=w1190, "Row Start"=w1189) -> ("Dielectric (d)"=w1194:dbl, "Index"=w1196:dbl, "XY Graph"=w1202:cluster{dbl[], dbl[]}[], "Length"=w1193:dbl, "Vt"=w1195:dbl, "Width"=w1170:dbl, "Table Control"=w1232:string[][], "Table Control 2"=w1231:string[][], "Recorded"=w1174:T6, "Mobility"=w1230:dbl)  [unwired: 2 in, 1 out]
            n397 = local write "Dielectric (d)"(w1194) -> ()
            n398 = local write "New Dielectric"(w1194) -> ()
            n399 = local write "New Length"(w1193) -> ()
            n400 = local write "New Width"(w1170) -> ()
            n401 = local write "Table Control"(w1232) -> ()
            n402 = Decimate 1D Array(w1202) -> (w1203:cluster{dbl[], dbl[]}[])  [unwired: 1 out]
            n403 = local write "XY Graph 2"(w1179) -> ()
            n404 = Array To Cluster(array=w1203) -> (cluster=w1205:T5)
            n405 = local write "XY Graph"(w1202) -> ()
            n406 = local write "Index 2"(w1183) -> ()
            n407 = local write "Table Control 2"(w1231) -> ()
            n408 = local write "Mobility"(w1230) -> ()
            n409 = local write "Length"(w1193) -> ()
            n410 = Unbundle(w1205) -> ("[0]"=w1204:cluster{dbl[], dbl[]})  [unwired: 8 out]
            n411 = Unbundle(w1204) -> (w1188:dbl[], w1187:dbl[])
            n412 = local write "Threshold V"(w1195) -> ()
            n413 = local write "Width"(w1170) -> ()
            n414 = Unbundle(w1174) -> ("Vt"=w1176:dbl, "STS"=w1175:dbl, "On/Off"=w1173:dbl)  [unwired: 4 out]
            n415 = Array Subset(array=w1188, index=w1196, length=w1190) -> (w1201:dbl[])
            n416 = Array Subset(array=w1187, index=w1196, length=w1190) -> (w1200:dbl[])
            n417 = local write "STS recorded"(w1175) -> ()
            n418 = local write "Data File"(w1191) -> ()
            n419 = local write "Index"(w1196) -> ()
            n420 = local write "Vt recorded"(w1176) -> ()
            n421 = local write "On/Off"(w1173) -> ()
            n422 = local write "Array 2"(w1200) -> ()
            n423 = local write "Array"(w1201) -> ()
            n424 = local read "Image Folder"() -> (w1162:path)
            n425 = local write "Slide"(w1196) -> ()
            n426 = List Folder(path=w1162, error in=w1158) -> (filenames=w1213:string[], error out=w1157:errorcluster)  [unwired: 2 in, 2 out]
            n427 = call-poly <vilib>:"Read From Spreadsheet File.vi"("file path (dialog if empty)"=w1191) -> ("all rows"=w1221:string[][])  [unwired: 6 in, 4 out]
            n428 = Array Size(array=w1221) -> (size(s)=w1220:i32[])
            n429 = Index Array(array=w1220, index=w1219) -> (element=w1198:i32)
            n430 = Subtract(x=w1198, y=20) -> (x-y=w1197:i32)
            n431 = property on="Slide" class="Slide (strict)"("Scale.Maximum"=w1197) -> ()  [unwired: 2 in, 2 out]
            n432 = Array Subset(array=w1221, index (row)=w1219, index (col)=w1219, length (col)=3) -> (w1222:string[][])  [unwired: 1 in]
            n433 = Reshape Array(w1222, w1198) -> (w1208:string[])
            n434 = Search 1D Array(1D array=w1208, element="Mobility (cm^2/Vs):") -> (index of element=w1211:i32)  [unwired: 1 in]
            n435 = Increment(x=w1211) -> (x+1=w1210:i32)
            n436 = Index Array(array=w1208, index=w1210) -> (element=w1207:string)
            n437 = Fract/Exp String To Number(string=w1207) -> (number=w1206:dbl)  [unwired: 3 in, 1 out]
            n438 = local write "Recorded Mobility"(w1206) -> ()
            n439 = Search 1D Array(1D array=w1208, element="Index:") -> (index of element=w1216:i32)  [unwired: 1 in]
            n440 = Increment(x=w1216) -> (x+1=w1217:i32)
            n441 = Index Array(array=w1208, index=w1217) -> (element=w1154:string)
            n442 = while {
              tunnel: w1213 -> [w1249]
              tunnel: w1154 -> [w1247]
              tunnel: [w1246] -> w1212
              tunnel: w1198 -> [w1245]
              i -> [w1246]
              stop <- w1242 stop-if-true
              n443 = Index Array(array=w1249, index=w1246) -> (element=w1250:string)
              n444 = xnode "Match Regular Expression"("input string"=w1250, "regular expression"=w1247) -> ("whole match"=w1248:string)  [unwired: 4 in, 4 out]
              n445 = Equal?(x=w1248, y=w1247) -> (x = y?=w1244:bool)
              n446 = Equal?(x=w1245, y=w1246) -> (x = y?=w1243:bool)
              n447 = Or(x=w1244, y=w1243) -> (x .or. y?=w1242:bool)
            }
            n448 = local write "Index 3"(w1154) -> ()
            n449 = Build Path(base path=w1162, name or relative path="ROI") -> (appended path=w1155:path)
            n450 = Build Path(base path=w1155, name or relative path=w1154) -> (appended path=w1153:path)
            n451 = invoke on="Image Out" class="ImageControl" method="Clear ROI"(error in=w1157) -> (error out=w1161:errorcluster)  [unwired: 2 in, 2 out]
            n452 = call <vilib>:"Check if File or Folder Exists.vi"("error in (no error)"=w1161, "path"=w1153) -> ("file or folder exists?"=w1159:bool, "dup path"=w1160:path)  [unwired: 7 in, 1 out]
            n453 = local read "No Image"() -> (w1171:path)
            n454 = Index Array(array=w1213, index=w1212) -> (element=w1164:string)
            n455 = Build Path(base path=w1162, name or relative path=w1164) -> (appended path=w1163:path)
            n456 = local write "Image Name"(w1164) -> ()
            n457 = Empty String/Path?(string/path=w1164) -> (empty?=w1172:bool)
            n458 = case shown="True" w1159 {
              tunnel: w1160 -> [_ w1237]
              frame False {
              }
              frame True {
                n459 = Read from Text File(file (use dialog)=w1237) -> (text=w1241:string)  [unwired: 3 in, 3 out]
                n460 = property on="Image Out" class="ImageControl"() -> ("ROI"=w1238:T7)  [unwired: 2 in, 2 out]
                n461 = Unflatten From String(type=w1238, binary string=w1241) -> (value=w1239:T7, error out=w1240:errorcluster)  [unwired: 3 in, 1 out]
                n462 = property on="Image Out" class="ImageControl"(error in=w1240, "ROI"=w1239) -> ()  [unwired: 1 in, 2 out]
              }
            }
            n463 = Select(t=w1171, s=w1172, f=w1163) -> (s? t:f=w1165:path)
            n464 = call "Vision Acquisition5"("Image Path"=w1165) -> ("Image Out"=w1169:T2)  [unwired: 25 in, 1 out]
            n465 = local write "Image File"(w1165) -> ()
            n466 = local write "Image Out 2"(w1169) -> ()
            n467 = local write "Image Out"(w1169) -> ()
            n468 = call <vilib>:"Get File Extension.vi"("file"=w1165) -> ("lowercase file extension"=w1167:string)  [unwired: 7 in, 3 out]
            n469 = local write "String"(w1167) -> ()
            n470 = Search 1D Array(1D array=string[] ["bmp", "jpeg", "png", "jpg", "gif"], element=w1167) -> (index of element=w1166:i32)  [unwired: 1 in]
            n471 = Less Than 0?(x=w1166) -> ()  [unwired: 1 out]
          }
          event "Save Changes? 3": Mouse Down {
            n472 = event-data() -> ()  [unwired: 1 in, 7 out]
            n473 = local read "Image Folder"() -> (w1366:path)
            n474 = Build Path(base path=w1366, name or relative path="ROI") -> (appended path=w1373:path)
            n475 = call <vilib>:"Check if File or Folder Exists.vi"("path"=w1373) -> ("file or folder exists?"=w1375:bool, "dup path"=w1372:path)  [unwired: 8 in, 1 out]
            n476 = case shown="False" w1375 {
              tunnel: w1372 -> [w1377 w1378]
              tunnel: [w1376 w1378] -> w1367
              frame False {
                n477 = Create Folder(path (use dialog)=w1377) -> (created path=w1376:path)  [unwired: 2 in, 2 out]
              }
              frame True {
              }
            }
            n478 = property on="Image Out" class="ImageControl"() -> ("ROI"=w1371:T7)  [unwired: 2 in, 2 out]
            n479 = local read "Index 3"() -> (w1369:string)
            n480 = Flatten To String(anything=w1371) -> (data string=w1370:string)  [unwired: 3 in, 2 out]
            n481 = Build Path(base path=w1367, name or relative path=w1369) -> (appended path=w1368:path)
            n482 = Write to Text File(file (use dialog)=w1368, text=w1370) -> ()  [unwired: 2 in, 3 out]
          }
          event "Next Button": Mouse Down {
            n483 = event-data() -> ()  [unwired: 1 in, 5 out]
            n484 = local read "XY Graph"() -> (w1391:cluster{dbl[], dbl[]}[])
            n485 = local read "NumPts"() -> (w1392:dbl)
            n486 = local read "Index"() -> (w1393:dbl)
            n487 = Decimate 1D Array(w1391) -> (w1387:cluster{dbl[], dbl[]}[], w1386:cluster{dbl[], dbl[]}[])
            n488 = Array To Cluster(array=w1387) -> (cluster=w1397:T5)
            n489 = Unbundle(w1397) -> ("[0]"=w1396:cluster{dbl[], dbl[]})  [unwired: 8 out]
            n490 = Increment(x=w1393) -> (x+1=w1388:dbl)
            n491 = Unbundle(w1396) -> (w1395:dbl[], w1394:dbl[])
            n492 = Array Subset(array=w1395, index=w1388, length=w1392) -> (w1384:dbl[])
            n493 = local write "Index"(w1388) -> ()
            n494 = Array Subset(array=w1394, index=w1388, length=w1392) -> (w1383:dbl[])
            n495 = Bundle(w1384, w1383) -> (w1390:cluster{dbl[], dbl[]})  [unwired: 1 in]
            n496 = Build Array (concatenate)(w1387, w1386, w1390) -> (w1389:cluster{dbl[], dbl[]}[])
            n497 = local write "XY Graph"(w1389) -> ()
            n498 = local read "New Dielectric"() -> (w1382:dbl)
            n499 = local write "Array 2"(w1383) -> ()
            n500 = local read "New Length"() -> (w1381:dbl)
            n501 = local write "Array"(w1384) -> ()
            n502 = local read "New Width"() -> (w1380:dbl)
            n503 = call "mob_calc_subvi.vi"("Width"=w1380, "Length"=w1381, "Dielectric (d)"=w1382, "Array 2"=w1383, "Array"=w1384) -> ("Vt"=w1379:dbl, "Mobility"=w1385:dbl)  [unwired: 5 in]
            n504 = local write "New Mobility"(w1385) -> ()
            n505 = local write "New Vt"(w1379) -> ()
          }
          event "Next Button 2": Mouse Down {
            n506 = event-data() -> ()  [unwired: 1 in, 7 out]
            n507 = local read "XY Graph 2"() -> (w1406:cluster{dbl[], dbl[]}[])
            n508 = local read "Index 2"() -> (w1408:dbl)
            n509 = local read "NumPts 2"() -> (w1407:dbl)
            n510 = Decimate 1D Array(w1406) -> (w1402:cluster{dbl[], dbl[]}[], w1401:cluster{dbl[], dbl[]}[])
            n511 = Array To Cluster(array=w1402) -> (cluster=w1412:T5)
            n512 = Unbundle(w1412) -> ("[0]"=w1411:cluster{dbl[], dbl[]})  [unwired: 8 out]
            n513 = Increment(x=w1408) -> (x+1=w1403:dbl)
            n514 = Unbundle(w1411) -> (w1410:dbl[], w1409:dbl[])
            n515 = local write "Index 2"(w1403) -> ()
            n516 = Array Subset(array=w1410, index=w1403, length=w1407) -> (w1399:dbl[])
            n517 = Array Subset(array=w1409, index=w1403, length=w1407) -> (w1398:dbl[])
            n518 = Bundle(w1399, w1398) -> (w1405:cluster{dbl[], dbl[]})  [unwired: 1 in]
            n519 = Build Array (concatenate)(w1402, w1401, w1405) -> (w1404:cluster{dbl[], dbl[]}[])
            n520 = local write "XY Graph 2"(w1404) -> ()
            n521 = local write "Array 8"(w1399) -> ()
            n522 = call "sts_calc_subvi.vi"("Array 2"=w1399, "Array"=w1398) -> ("STS"=w1400:dbl)  [unwired: 9 in]
            n523 = local write "Array 7"(w1398) -> ()
            n524 = local write "New S.T.S."(w1400) -> ()
          }
          event "Previous Button 2": Mouse Down {
            n525 = event-data() -> ()  [unwired: 1 in, 7 out]
            n526 = local read "XY Graph 2"() -> (w1422:cluster{dbl[], dbl[]}[])
            n527 = local read "NumPts 2"() -> (w1423:dbl)
            n528 = local read "Index 2"() -> (w1415:dbl)
            n529 = Decimate 1D Array(w1422) -> (w1419:cluster{dbl[], dbl[]}[], w1418:cluster{dbl[], dbl[]}[])
            n530 = Array To Cluster(array=w1419) -> (cluster=w1427:T5)
            n531 = Unbundle(w1427) -> ("[0]"=w1426:cluster{dbl[], dbl[]})  [unwired: 8 out]
            n532 = Decrement(x=w1415) -> (x-1=w1416:dbl)
            n533 = Unbundle(w1426) -> (w1425:dbl[], w1424:dbl[])
            n534 = local write "Index 2"(w1416) -> ()
            n535 = Array Subset(array=w1425, index=w1416, length=w1423) -> (w1413:dbl[])
            n536 = Array Subset(array=w1424, index=w1416, length=w1423) -> (w1414:dbl[])
            n537 = Bundle(w1413, w1414) -> (w1421:cluster{dbl[], dbl[]})  [unwired: 1 in]
            n538 = Build Array (concatenate)(w1419, w1418, w1421) -> (w1420:cluster{dbl[], dbl[]}[])
            n539 = local write "XY Graph 2"(w1420) -> ()
            n540 = local write "Array 7"(w1414) -> ()
            n541 = call "sts_calc_subvi.vi"("Array 2"=w1413, "Array"=w1414) -> ("STS"=w1417:dbl)  [unwired: 9 in]
            n542 = local write "Array 8"(w1413) -> ()
            n543 = local write "New S.T.S."(w1417) -> ()
          }
          event "Previous Button": Mouse Down {
            n544 = event-data() -> ()  [unwired: 1 in, 5 out]
            n545 = local read "XY Graph"() -> (w1441:cluster{dbl[], dbl[]}[])
            n546 = Decimate 1D Array(w1441) -> (w1438:cluster{dbl[], dbl[]}[], w1437:cluster{dbl[], dbl[]}[])
            n547 = local read "NumPts"() -> (w1442:dbl)
            n548 = local read "Index"() -> (w1436:dbl)
            n549 = Array To Cluster(array=w1438) -> (cluster=w1446:T5)
            n550 = Unbundle(w1446) -> ("[0]"=w1445:cluster{dbl[], dbl[]})  [unwired: 8 out]
            n551 = Decrement(x=w1436) -> (x-1=w1435:dbl)
            n552 = Unbundle(w1445) -> (w1444:dbl[], w1443:dbl[])
            n553 = local read "New Dielectric"() -> (w1429:dbl)
            n554 = Array Subset(array=w1444, index=w1435, length=w1442) -> (w1434:dbl[])
            n555 = Array Subset(array=w1443, index=w1435, length=w1442) -> (w1433:dbl[])
            n556 = local write "Index"(w1435) -> ()
            n557 = Bundle(w1434, w1433) -> (w1440:cluster{dbl[], dbl[]})  [unwired: 1 in]
            n558 = Build Array (concatenate)(w1438, w1437, w1440) -> (w1439:cluster{dbl[], dbl[]}[])
            n559 = local write "XY Graph"(w1439) -> ()
            n560 = local read "New Length"() -> (w1430:dbl)
            n561 = local write "Array 2"(w1433) -> ()
            n562 = local read "New Width"() -> (w1431:dbl)
            n563 = call "mob_calc_subvi.vi"("Width"=w1431, "Length"=w1430, "Dielectric (d)"=w1429, "Array 2"=w1433, "Array"=w1434) -> ("Vt"=w1428:dbl, "Mobility"=w1432:dbl)  [unwired: 5 in]
            n564 = local write "New Mobility"(w1432) -> ()
            n565 = local write "Array"(w1434) -> ()
            n566 = local write "New Vt"(w1428) -> ()
          }
          event "Slide": Value Change {
            n567 = event-data() -> ()  [unwired: 1 in, 5 out]
            n568 = local read "XY Graph"() -> (w1459:cluster{dbl[], dbl[]}[])
            n569 = local read "Slide"() -> (w1448:dbl)
            n570 = Decimate 1D Array(w1459) -> (w1456:cluster{dbl[], dbl[]}[], w1455:cluster{dbl[], dbl[]}[])
            n571 = local read "NumPts"() -> (w1460:dbl)
            n572 = Array To Cluster(array=w1456) -> (cluster=w1464:T5)
            n573 = Unbundle(w1464) -> ("[0]"=w1463:cluster{dbl[], dbl[]})  [unwired: 8 out]
            n574 = Unbundle(w1463) -> (w1462:dbl[], w1461:dbl[])
            n575 = local read "New Dielectric"() -> (w1449:dbl)
            n576 = Array Subset(array=w1462, index=w1448, length=w1460) -> (w1454:dbl[])
            n577 = Array Subset(array=w1461, index=w1448, length=w1460) -> (w1453:dbl[])
            n578 = local write "Index"(w1448) -> ()
            n579 = Bundle(w1454, w1453) -> (w1458:cluster{dbl[], dbl[]})  [unwired: 1 in]
            n580 = Build Array (concatenate)(w1456, w1455, w1458) -> (w1457:cluster{dbl[], dbl[]}[])
            n581 = local write "XY Graph"(w1457) -> ()
            n582 = local read "New Length"() -> (w1450:dbl)
            n583 = local write "Array 2"(w1453) -> ()
            n584 = local read "New Width"() -> (w1451:dbl)
            n585 = call "mob_calc_subvi.vi"("Width"=w1451, "Length"=w1450, "Dielectric (d)"=w1449, "Array 2"=w1453, "Array"=w1454) -> ("Vt"=w1447:dbl, "Mobility"=w1452:dbl)  [unwired: 5 in]
            n586 = local write "New Mobility"(w1452) -> ()
            n587 = local write "Array"(w1454) -> ()
            n588 = local write "New Vt"(w1447) -> ()
          }
          event "Slide 2": Value Change {
            n589 = event-data() -> ()  [unwired: 1 in, 5 out]
            n590 = local read "XY Graph 2"() -> (w1473:cluster{dbl[], dbl[]}[])
            n591 = local read "Slide 2"() -> (w1468:dbl)
            n592 = Decimate 1D Array(w1473) -> (w1470:cluster{dbl[], dbl[]}[], w1469:cluster{dbl[], dbl[]}[])
            n593 = local read "NumPts 2"() -> (w1474:dbl)
            n594 = Array To Cluster(array=w1470) -> (cluster=w1478:T5)
            n595 = Unbundle(w1478) -> ("[0]"=w1477:cluster{dbl[], dbl[]})  [unwired: 8 out]
            n596 = Unbundle(w1477) -> (w1476:dbl[], w1475:dbl[])
            n597 = Array Subset(array=w1476, index=w1468, length=w1474) -> (w1466:dbl[])
            n598 = Array Subset(array=w1475, index=w1468, length=w1474) -> (w1465:dbl[])
            n599 = local write "Index 2"(w1468) -> ()
            n600 = Bundle(w1466, w1465) -> (w1472:cluster{dbl[], dbl[]})  [unwired: 1 in]
            n601 = Build Array (concatenate)(w1470, w1469, w1472) -> (w1471:cluster{dbl[], dbl[]}[])
            n602 = local write "XY Graph 2"(w1471) -> ()
            n603 = local write "Array 7"(w1465) -> ()
            n604 = local write "Array 8"(w1466) -> ()
            n605 = call "sts_calc_subvi.vi"("Array 2"=w1466, "Array"=w1465) -> ("STS"=w1467:dbl)  [unwired: 9 in]
            n606 = local write "New S.T.S."(w1467) -> ()
          }
          event "Save Changes?": Mouse Down {
            w1516 = "/"
            n607 = event-data() -> ()  [unwired: 1 in, 5 out]
            n608 = local read "Date Recorded"() -> (w1513:string)
            n609 = local read "Index 3"() -> (w1569:string)
            n610 = Match Pattern(string=w1513, regular expression=w1516) -> (before substring=w1522:string, after substring=w1515:string)  [unwired: 1 in, 2 out]
            n611 = String Length(string=w1522) -> (length=w1519:i32)
            n612 = Match Pattern(string=w1515, regular expression=w1516) -> (before substring=w1528:string, after substring=w1517:string)  [unwired: 1 in, 2 out]
            n613 = Equal?(x=w1519, y=2) -> (x = y?=w1521:bool)
            n614 = String Subset(string=w1569, length (rest)=1) -> (substring=w1488:string)  [unwired: 1 in]
            n615 = local write "Row"(w1488) -> ()
            n616 = String Length(string=w1528) -> (length=w1526:i32)
            n617 = Equal?(x=w1526, y=2) -> (x = y?=w1524:bool)
            n618 = String Subset(string=w1569, offset (0)=1, length (rest)=2) -> (substring=w1487:string)
            n619 = case shown="False" w1524 {
              tunnel: w1528 -> [w1578 w1580]
              tunnel: [w1577 w1580] -> w1527
              frame False {
                n620 = Concatenate Strings("0", w1578) -> (w1577:string)
              }
              frame True {
              }
            }
            n621 = case shown="False" w1521 {
              tunnel: w1522 -> [w1582 w1584]
              tunnel: [w1581 w1584] -> w1523
              frame False {
                n622 = Concatenate Strings("0", w1582) -> (w1581:string)
              }
              frame True {
              }
            }
            n623 = Build Array("DeviceID", "Fabricator", "Deposition", "Date", "Sample", "Row", "Column", "L (um)", "W (um)", "Material", "Treatment", "TC (mM)", "Solvent", "C (%)", "ST (C)", "Drops", "Wait (s)", "RT (F)", "RH (%)", "Ramp (s)", "RPM", "Accel (RPM/s)", "Time (s)", "Mobility", "On/Off", "Vt", "S.T.S") -> (w1485:string[])
            n624 = local write "Column"(w1487) -> ()
            n625 = local read "Index 3"() -> (w1529:string)
            n626 = local write "Transformer \nHeaders"(w1485) -> ()
            n627 = local read "Wait Time (s):"() -> (w1480:dbl)
            n628 = local read "Treatment Concentration (mM):"() -> (w1536:dbl)
            n629 = local read "Relative Humidity (%):"() -> (w1539:dbl)
            n630 = Number To Decimal String(number=w1480) -> (decimal integer string=w1479:string)  [unwired: 1 in]
            n631 = local read "Solution Temp (C):"() -> (w1494:dbl)
            n632 = local read "Surface Treatment:"() -> (w1537:string)
            n633 = local read "Material Recorded"() -> (w1541:string)
            n634 = local read "Room Temp (F):"() -> (w1490:dbl)
            n635 = local read "Concentration Recorded"() -> (w1534:string)
            n636 = local read "New Length"() -> (w1530:dbl)
            n637 = local read "New Width"() -> (w1531:dbl)
            n638 = local read "Accel (RPM/s):"() -> (w1503:dbl)
            n639 = local read "Sample #:"() -> (w1511:dbl)
            n640 = local read "New Mobility"() -> (w1501:dbl)
            n641 = local read "Method Recorded"() -> (w1510:string)
            n642 = local read "# Drops:"() -> (w1493:dbl)
            n643 = local read "Ramp (s):"() -> (w1483:dbl)
            n644 = local read "Solvent Recorded"() -> (w1535:string)
            n645 = local read "New S.T.S."() -> (w1509:dbl)
            n646 = local read "Date Recorded"() -> (w1514:string)
            n647 = local read "Time (s):"() -> (w1498:dbl)
            n648 = local read "On/Off"() -> (w1505:dbl)
            n649 = local read "New Vt"() -> (w1507:dbl)
            n650 = local read "RPM:"() -> (w1497:dbl)
            n651 = local read "Fabricator:"() -> (w1489:string)
            n652 = Number To Decimal String(number=w1493) -> (decimal integer string=w1492:string)  [unwired: 1 in]
            n653 = Number To Decimal String(number=w1511) -> (decimal integer string=w1518:string)  [unwired: 1 in]
            n654 = call "DeviceID"("Sample"=w1518, "Year"=w1517, "Month"=w1523, "Day"=w1527, "Index"=w1529) -> ("Result"=w1512:string)  [unwired: 9 in, 1 out]
            n655 = Number To Decimal String(number=w1530) -> (decimal integer string=w1532:string)  [unwired: 1 in]
            n656 = Number To Decimal String(number=w1531) -> (decimal integer string=w1533:string)  [unwired: 1 in]
            n657 = Number To Decimal String(number=w1494) -> (decimal integer string=w1495:string)  [unwired: 1 in]
            n658 = Number To Decimal String(number=w1539) -> (decimal integer string=w1540:string)  [unwired: 1 in]
            n659 = Number To Decimal String(number=w1490) -> (decimal integer string=w1491:string)  [unwired: 1 in]
            n660 = Number To Decimal String(number=w1536) -> (decimal integer string=w1538:string)  [unwired: 1 in]
            n661 = Number To Decimal String(number=w1497) -> (decimal integer string=w1496:string)  [unwired: 1 in]
            n662 = Number To Fractional String(number=w1503) -> (F-format string=w1502:string)  [unwired: 3 in]
            n663 = Number To Decimal String(number=w1498) -> (decimal integer string=w1499:string)  [unwired: 1 in]
            n664 = Number To Fractional String(number=w1501) -> (F-format string=w1500:string)  [unwired: 3 in]
            n665 = Number To Fractional String(number=w1505) -> (F-format string=w1504:string)  [unwired: 3 in]
            n666 = Number To Fractional String(number=w1507) -> (F-format string=w1506:string)  [unwired: 3 in]
            n667 = Number To Fractional String(number=w1509) -> (F-format string=w1508:string)  [unwired: 3 in]
            n668 = Number To Decimal String(number=w1483) -> (decimal integer string=w1482:string)  [unwired: 1 in]
            n669 = Build Array(w1512, w1489, w1510, w1514, w1518, w1488, w1487, w1532, w1533, w1541, w1537, w1538, w1535, w1534, w1495, w1492, w1479, w1491, w1540, w1482, w1496, w1502, w1499, w1500, w1504, w1506, w1508) -> (w1486:string[])
            n670 = local write "Current \nRecord"(w1486) -> ()
            n671 = flat-sequence {
              tunnel: [w1606] -> w1576
              tunnel: [w1605] -> w1574
              tunnel: [w1605] -> w1573
              tunnel: [w1588] -> w1571
              tunnel: w1576 -> [w1714]
              tunnel: [w1715] -> w1575
              tunnel: w1574 -> [w1715]
              tunnel: w1573 -> [w1713]
              tunnel: [w1711] -> w1572
              tunnel: w1571 -> [w1711]
              tunnel: w1575 -> [w1720]
              tunnel: w1572 -> [w1719]
              frame #0 {
                w1593 = -1
                w1586 = "S.T.S. (V/decade):"
                w1587 = "Threshold V (V):"
                (unwired) 3
                w1591 = 1
                n672 = local read "Data File"() -> (w1606:path)
                n673 = local read "New Dielectric"() -> (w1629:dbl)
                n674 = local read "New Width"() -> (w1619:dbl)
                n675 = local read "New Length"() -> (w1617:dbl)
                n676 = local read "New Mobility"() -> (w1628:dbl)
                n677 = flat-sequence {
                  tunnel: [w1642] -> w1585
                  tunnel: w1585 -> [w1659]
                  frame #0 {
                    # "Makes Empty File for Transformer Data"
                    n678 = local read "Data Folder"() -> (w1631:path)
                    n679 = Build Path(base path=w1631, name or relative path="Stats") -> (appended path=w1633:path)
                    n680 = call <vilib>:"Check if File or Folder Exists.vi"("path"=w1633) -> ("file or folder exists?"=w1634:bool, "dup path"=w1635:path)  [unwired: 8 in, 1 out]
                    n681 = case shown="False" w1634 {
                      tunnel: [w1639 w1641] -> w1636
                      tunnel: w1635 -> [w1640 w1641]
                      frame False {
                        n682 = Create Folder(path (use dialog)=w1640) -> (created path=w1639:path)  [unwired: 2 in, 2 out]
                      }
                      frame True {
                      }
                    }
                    n683 = Build Path(base path=w1636, name or relative path="Tranformer Data.txt") -> (appended path=w1638:path)
                    n684 = call-poly <vilib>:"Write To Spreadsheet File.vi"("append to file? (new file:F)"=TRUE, "file path (dialog if empty)"=w1638) -> ()  [unwired: 6 in, 1 out]
                  }
                  frame #1 {
                    # "Adds Headers if they don't exist"
                    n685 = Concatenate Strings("Stats\\", "Tranformer Data.txt") -> (w1649:string)
                    n686 = local read "Data Folder"() -> (w1648:path)
                    n687 = Build Path(base path=w1648, name or relative path=w1649) -> (appended path=w1642:path)
                    n688 = call-poly <vilib>:"Read From Spreadsheet File.vi"("file path (dialog if empty)"=w1642) -> ("first row"=w1647:string[])  [unwired: 6 in, 4 out]
                    n689 = Search 1D Array(1D array=w1647, element="DeviceID") -> (index of element=w1645:i32)  [unwired: 1 in]
                    n690 = Equal?(x=w1645, y=0) -> (x = y?=w1643:bool)
                    n691 = case shown="False" w1643 {
                      tunnel: w1642 -> [w1653 _]
                      frame False {
                        n692 = local read "Transformer \nHeaders"() -> (w1652:string[])
                        n693 = call-poly <vilib>:"Write To Spreadsheet File.vi"("1D data"=w1652, "file path (dialog if empty)"=w1653) -> ()  [unwired: 6 in, 1 out]
                      }
                      frame True {
                      }
                    }
                  }
                  frame #2 {
                    # "Adds current device if it doesn't exist"
                    n694 = local read "Current \nRecord"() -> (w1658:string[])
                    n695 = Index Array(array=w1658, index=0) -> (element=w1657:string)
                    n696 = Concatenate Strings("Stats\\", "Tranformer Data.txt") -> (w1662:string)
                    n697 = local read "Data Folder"() -> (w1661:path)
                    n698 = local write "Current Device ID"(w1657) -> ()
                    n699 = local read "Current Device ID"() -> (w1667:string)
                    n700 = Build Path(base path=w1661, name or relative path=w1662) -> (appended path=w1660:path)
                    n701 = call-poly <vilib>:"Read From Spreadsheet File.vi"("file path (dialog if empty)"=w1660) -> ("all rows"=w1654:string[][])  [unwired: 6 in, 4 out]
                    n702 = Index Array(array=w1654, index (col)=0) -> (element=w1655:string[])  [unwired: 1 in]
                    n703 = Search 1D Array(1D array=w1655, element=w1667) -> (index of element=w1656:i32)  [unwired: 1 in]
                    n704 = Equal?(x=w1656, y=-1) -> (x = y?=w1669:bool)
                    n705 = case shown="False" w1669 {
                      tunnel: w1659 -> [w1672 w1683]
                      tunnel: w1656 -> [w1675 _]
                      tunnel: w1654 -> [w1676 _]
                      frame False {
                        n706 = local read "Current \nRecord"() -> (w1674:string[])
                        n707 = Replace Array Subset(array=w1676, new element=w1674, index (row)=w1675) -> (w1673:string[][])  [unwired: 1 in]
                        n708 = flat-sequence {
                          tunnel: w1672 -> [w1677]
                          tunnel: w1673 -> [w1678]
                          tunnel: [w1678] -> w1671
                          tunnel: [w1677] -> w1670
                          tunnel: w1671 -> [w1680]
                          tunnel: w1670 -> [w1679]
                          frame #0 {
                            n709 = Delete(path (use dialog)=w1677) -> ()  [unwired: 4 in, 3 out]
                          }
                          frame #1 {
                            n710 = call-poly <vilib>:"Write To Spreadsheet File.vi"("append to file? (new file:F)"=TRUE, "2D data"=w1680, "file path (dialog if empty)"=w1679) -> ()  [unwired: 5 in, 1 out]
                          }
                        }
                      }
                      frame True {
                        n711 = local read "Current \nRecord"() -> (w1682:string[])
                        n712 = call-poly <vilib>:"Write To Spreadsheet File.vi"("append to file? (new file:F)"=TRUE, "1D data"=w1682, "file path (dialog if empty)"=w1683) -> ()  [unwired: 5 in, 1 out]
                      }
                    }
                  }
                }
                n713 = call-poly <vilib>:"Read From Spreadsheet File.vi"("file path (dialog if empty)"=w1606) -> ("all rows"=w1598:string[][])  [unwired: 6 in, 4 out]
                n714 = Number To Fractional String(number=w1617) -> (F-format string=w1609:string)  [unwired: 3 in]
                n715 = Replace Array Subset(array=w1598, new element=w1609, index (row)=12, index (col)=w1591) -> (w1613:string[][])
                n716 = Number To Fractional String(number=w1619) -> (F-format string=w1620:string)  [unwired: 3 in]
                n717 = Replace Array Subset(array=w1613, new element=w1620, index (row)=13, index (col)=w1591) -> (w1615:string[][])
                n718 = Number To Fractional String(number=w1628) -> (F-format string=w1607:string)  [unwired: 3 in]
                n719 = Number To Fractional String(number=w1629) -> (F-format string=w1608:string)  [unwired: 3 in]
                n720 = Number To Decimal String(number=w1617) -> (decimal integer string=w1616:string)  [unwired: 1 in]
                n721 = Strip Path(path=w1606) -> (stripped path=w1627:path)  [unwired: 1 out]
                n722 = local read "Index 3"() -> (w1622:string)
                n723 = Replace Array Subset(array=w1615, new element=w1607, index (row)=15, index (col)=w1591) -> (w1614:string[][])
                n724 = Number To Decimal String(number=w1619) -> (decimal integer string=w1618:string)  [unwired: 1 in]
                n725 = Path To String(path=w1627) -> (string=w1625:string)
                n726 = Replace Array Subset(array=w1614, new element=w1608, index (row)=7, index (col)=w1591) -> (w1590:string[][])
                n727 = call "Build Text"("Index"=w1622, "Length"=w1616, "Width"=w1618) -> ("Result"=w1623:string)  [unwired: 11 in, 1 out]
                n728 = Concatenate Strings(w1625, "\\", w1623) -> (w1624:string)
                n729 = String To Path(string=w1624) -> (path=w1605:path)
                n730 = Array Size(array=w1598) -> (size(s)=w1600:i32[])
                n731 = Index Array(array=w1600, index=0) -> (element=w1599:i32)
                n732 = Array Subset(array=w1598, index (row)=0, index (col)=0) -> (w1604:string[][])  [unwired: 2 in]
                n733 = Reshape Array(w1604, w1599) -> (w1592:string[])
                n734 = Search 1D Array(1D array=w1592, element=w1587) -> (index of element=w1596:i32)  [unwired: 1 in]
                n735 = Search 1D Array(1D array=w1592, element=w1586) -> (index of element=w1597:i32)  [unwired: 1 in]
                n736 = Equal?(x=w1596, y=w1593) -> (x = y?=w1594:bool)
                n737 = Equal?(x=w1597, y=w1593) -> (x = y?=w1595:bool)
                n738 = case shown="True" w1594 {
                  tunnel: w1596 -> [_ _]
                  tunnel: w1590 -> [w1701 w1709]
                  tunnel: [w1700 w1708] -> w1589
                  tunnel: w1587 -> [_ w1707]
                  frame False {
                    n739 = local read "New Vt"() -> (w1703:dbl)
                    n740 = Number To Fractional String(number=w1703) -> (F-format string=w1699:string)  [unwired: 3 in]
                    n741 = Replace Array Subset(array=w1701, new element=w1699, index (row)=17, index (col)=1) -> (w1700:string[][])
                  }
                  frame True {
                    n742 = local read "New Vt"() -> (w1710:dbl)
                    n743 = Number To Fractional String(number=w1710) -> (F-format string=w1706:string)  [unwired: 3 in]
                    n744 = Build Array(w1707, w1706) -> (w1705:string[])
                    n745 = Insert Into Array(array=w1709, index (row)=17, new element=w1705) -> (w1708:string[][])  [unwired: 1 in]
                  }
                }
                n746 = case shown="True" w1595 {
                  tunnel: w1597 -> [_ _]
                  tunnel: w1589 -> [w1688 w1696]
                  tunnel: [w1687 w1695] -> w1588
                  tunnel: w1586 -> [_ w1693]
                  frame False {
                    n747 = local read "New S.T.S."() -> (w1690:dbl)
                    n748 = Number To Fractional String(number=w1690) -> (F-format string=w1686:string)  [unwired: 3 in]
                    n749 = Replace Array Subset(array=w1688, new element=w1686, index (row)=18, index (col)=1) -> (w1687:string[][])
                  }
                  frame True {
                    n750 = local read "New S.T.S."() -> (w1697:dbl)
                    n751 = Number To Fractional String(number=w1697) -> (F-format string=w1694:string)  [unwired: 3 in]
                    n752 = Build Array(w1693, w1694) -> (w1692:string[])
                    n753 = Insert Into Array(array=w1696, index (row)=18, new element=w1692) -> (w1695:string[][])  [unwired: 1 in]
                  }
                }
              }
              frame #1 {
                n754 = Equal?(x=w1714, y=w1713) -> (x = y?=w1712:bool)
                n755 = case shown="False" w1712 {
                  tunnel: w1714 -> [w1718 _]
                  tunnel: w1713 -> [w1717 _]
                  frame False {
                    n756 = Move(source path=w1718, 9:TRUE, 10:w1717) -> ()  [unwired: 2 in, 3 out]
                  }
                  frame True {
                  }
                }
              }
              frame #2 {
                n757 = local write "Data File"(w1720) -> ()
                n758 = call-poly <vilib>:"Write To Spreadsheet File.vi"("2D data"=w1719, "file path (dialog if empty)"=w1720) -> ()  [unwired: 6 in, 1 out]
              }
            }
          }
          event "Save Changes? 2": Mouse Down {
            n759 = event-data() -> ()  [unwired: 1 in, 5 out]
            n760 = stacked-sequence {
              seq-local: [w1797 _ _ _ _ _] -> [_ w1850 _ _ _ _]
              seq-local: [w1796 _ _ _ _ _] -> [_ w1851 _ _ _ _]
              seq-local: [w1796 _ _ _ _ _] -> [_ w1849 _ _ _ _]
              seq-local: [w1779 _ _ _ _ _] -> [_ w1847 _ _ _ _]
              seq-local: [_ w1851 _ _ _ _] -> [_ _ w1856 _ _ _]
              seq-local: [_ w1847 _ _ _ _] -> [_ _ w1855 _ _ _]
              frame #0 {
                w1784 = -1
                w1777 = "S.T.S. (V/decade):"
                w1778 = "Threshold V (V):"
                (unwired) 3
                w1782 = 1
                n761 = local read "Data File"() -> (w1797:path)
                n762 = local read "New Width"() -> (w1810:dbl)
                n763 = local read "New Dielectric"() -> (w1820:dbl)
                n764 = local read "New Length"() -> (w1808:dbl)
                n765 = local read "New Mobility"() -> (w1819:dbl)
                n766 = call-poly <vilib>:"Read From Spreadsheet File.vi"("file path (dialog if empty)"=w1797) -> ("all rows"=w1789:string[][])  [unwired: 6 in, 4 out]
                n767 = Number To Fractional String(number=w1808) -> (F-format string=w1800:string)  [unwired: 3 in]
                n768 = Replace Array Subset(array=w1789, new element=w1800, index (row)=12, index (col)=w1782) -> (w1804:string[][])
                n769 = Number To Fractional String(number=w1810) -> (F-format string=w1811:string)  [unwired: 3 in]
                n770 = Replace Array Subset(array=w1804, new element=w1811, index (row)=13, index (col)=w1782) -> (w1806:string[][])
                n771 = Number To Fractional String(number=w1819) -> (F-format string=w1798:string)  [unwired: 3 in]
                n772 = Number To Fractional String(number=w1820) -> (F-format string=w1799:string)  [unwired: 3 in]
                n773 = Number To Decimal String(number=w1808) -> (decimal integer string=w1807:string)  [unwired: 1 in]
                n774 = Strip Path(path=w1797) -> (stripped path=w1818:path)  [unwired: 1 out]
                n775 = local read "Index 3"() -> (w1813:string)
                n776 = Replace Array Subset(array=w1806, new element=w1798, index (row)=15, index (col)=w1782) -> (w1805:string[][])
                n777 = Number To Decimal String(number=w1810) -> (decimal integer string=w1809:string)  [unwired: 1 in]
                n778 = Path To String(path=w1818) -> (string=w1816:string)
                n779 = Replace Array Subset(array=w1805, new element=w1799, index (row)=7, index (col)=w1782) -> (w1781:string[][])
                n780 = call "Build Text2"("Index"=w1813, "Length"=w1807, "Width"=w1809) -> ("Result"=w1814:string)  [unwired: 11 in, 1 out]
                n781 = Concatenate Strings(w1816, "\\", w1814) -> (w1815:string)
                n782 = String To Path(string=w1815) -> (path=w1796:path)
                n783 = Array Size(array=w1789) -> (size(s)=w1791:i32[])
                n784 = Index Array(array=w1791, index=0) -> (element=w1790:i32)
                n785 = Array Subset(array=w1789, index (row)=0, index (col)=0) -> (w1795:string[][])  [unwired: 2 in]
                n786 = Reshape Array(w1795, w1790) -> (w1783:string[])
                n787 = Search 1D Array(1D array=w1783, element=w1778) -> (index of element=w1787:i32)  [unwired: 1 in]
                n788 = Search 1D Array(1D array=w1783, element=w1777) -> (index of element=w1788:i32)  [unwired: 1 in]
                n789 = Equal?(x=w1787, y=w1784) -> (x = y?=w1785:bool)
                n790 = Equal?(x=w1788, y=w1784) -> (x = y?=w1786:bool)
                n791 = case shown="True" w1785 {
                  tunnel: w1787 -> [_ _]
                  tunnel: w1781 -> [w1837 w1845]
                  tunnel: [w1836 w1844] -> w1780
                  tunnel: w1778 -> [_ w1843]
                  frame False {
                    n792 = local read "New Vt"() -> (w1839:dbl)
                    n793 = Number To Fractional String(number=w1839) -> (F-format string=w1835:string)  [unwired: 3 in]
                    n794 = Replace Array Subset(array=w1837, new element=w1835, index (row)=17, index (col)=1) -> (w1836:string[][])
                  }
                  frame True {
                    n795 = local read "New Vt"() -> (w1846:dbl)
                    n796 = Number To Fractional String(number=w1846) -> (F-format string=w1842:string)  [unwired: 3 in]
                    n797 = Build Array(w1843, w1842) -> (w1841:string[])
                    n798 = Insert Into Array(array=w1845, index (row)=17, new element=w1841) -> (w1844:string[][])  [unwired: 1 in]
                  }
                }
                n799 = case shown="True" w1786 {
                  tunnel: w1788 -> [_ _]
                  tunnel: w1780 -> [w1824 w1832]
                  tunnel: [w1823 w1831] -> w1779
                  tunnel: w1777 -> [_ w1829]
                  frame False {
                    n800 = local read "New S.T.S."() -> (w1826:dbl)
                    n801 = Number To Fractional String(number=w1826) -> (F-format string=w1822:string)  [unwired: 3 in]
                    n802 = Replace Array Subset(array=w1824, new element=w1822, index (row)=18, index (col)=1) -> (w1823:string[][])
                  }
                  frame True {
                    n803 = local read "New S.T.S."() -> (w1833:dbl)
                    n804 = Number To Fractional String(number=w1833) -> (F-format string=w1830:string)  [unwired: 3 in]
                    n805 = Build Array(w1829, w1830) -> (w1828:string[])
                    n806 = Insert Into Array(array=w1832, index (row)=18, new element=w1828) -> (w1831:string[][])  [unwired: 1 in]
                  }
                }
              }
              frame #1 {
                n807 = Equal?(x=w1850, y=w1849) -> (x = y?=w1848:bool)
                n808 = case shown="False" w1848 {
                  tunnel: w1850 -> [w1854 _]
                  tunnel: w1849 -> [w1853 _]
                  frame False {
                    n809 = Move(source path=w1854, 9:TRUE, 10:w1853) -> ()  [unwired: 2 in, 3 out]
                  }
                  frame True {
                  }
                }
              }
              frame #2 {
                n810 = local write "Data File"(w1856) -> ()
                n811 = call-poly <vilib>:"Write To Spreadsheet File.vi"("2D data"=w1855, "file path (dialog if empty)"=w1856) -> ()  [unwired: 6 in, 1 out]
              }
              frame #3 {
                w1920 = 0
                n812 = local read "NumPts 2"() -> (w1879:dbl)
                n813 = local read "NumPts"() -> (w1886:dbl)
                n814 = local read "Row Start"() -> (w1885:dbl)
                n815 = local read "Data File"() -> (w1925:path)
                n816 = property on="Image Out" class="ImageControl"() -> (error out=w1860:errorcluster, "Image Center Position"=w1864:cluster{"X":u32, "Y":u32})  [unwired: 2 in, 1 out]
                n817 = Strip Path(path=w1925) -> (stripped path=w1916:path, name=w1938:string)
                n818 = local write "Data Folder"(w1916) -> ()
                n819 = List Folder(path=w1916) -> (filenames=w1931:string[])  [unwired: 3 in, 3 out]
                n820 = Unbundle(w1864) -> ("X"=w1862:u32)  [unwired: 1 out]
                n821 = Array Size(array=w1931) -> (size(s)=w1926:i32)
                n822 = Path To String(path=w1916) -> (string=w1939:string)
                n823 = Search 1D Array(1D array=w1931, element=w1938) -> (index of element=w1928:i32)  [unwired: 1 in]
                n824 = Bundle("X"=w1862, 0) -> (w1863:cluster{"X":u32, i32})  [unwired: 1 in]
                n825 = Decrement(x=w1926) -> (x-1=w1929:i32)
                n826 = Equal?(x=w1928, y=w1929) -> (x = y?=w1930:bool)
                n827 = case shown="False" w1930 {
                  tunnel: w1928 -> [w2061 _]
                  tunnel: [w2060 0] -> w1927
                  frame False {
                    n828 = Increment(x=w2061) -> (x+1=w2060:i32)
                  }
                  frame True {
                  }
                }
                n829 = Index Array(array=w1931, index=w1927) -> (element=w1932:string)
                n830 = local write "Data Name"(w1932) -> ()
                n831 = Concatenate Strings(w1939, "\\", w1932) -> (w1937:string)
                n832 = property on="Image Out" class="ImageControl"(error in=w1860, "Image Center Position"=w1863) -> ()  [unwired: 1 in, 2 out]
                n833 = String To Path(string=w1937) -> (path=w1887:path)
                n834 = call "sub_thresh_swing_subvi.vi"("Path"=w1887, "NumPts"=w1879, "Row Start"=w1885) -> ("Index"=w1880:dbl, "XY Graph"=w1875:cluster{dbl[], dbl[]}[], "Sub Threshold Swing"=w1888:dbl)  [unwired: 8 in, 2 out]
                n835 = Decimate 1D Array(w1875) -> (w1878:cluster{dbl[], dbl[]}[])  [unwired: 1 out]
                n836 = Array To Cluster(array=w1878) -> (cluster=w1876:T5)
                n837 = Unbundle(w1876) -> ("[0]"=w1877:cluster{dbl[], dbl[]})  [unwired: 8 out]
                n838 = Unbundle(w1877) -> (w1874:dbl[], w1873:dbl[])
                n839 = local write "S.T.S."(w1888) -> ()
                n840 = local write "XY Graph 2"(w1875) -> ()
                n841 = local write "Index 2"(w1880) -> ()
                n842 = call "mobility_subvi.vi"("Path"=w1887, "NumPts"=w1886, "Row Start"=w1885) -> ("Dielectric (d)"=w1891:dbl, "Index"=w1896:dbl, "XY Graph"=w1899:cluster{dbl[], dbl[]}[], "Length"=w1889:dbl, "Vt"=w1892:dbl, "Width"=w1890:dbl, "Table Control"=w1935:string[][], "Table Control 2"=w1934:string[][], "Recorded"=w1872:T6, "Mobility"=w1933:dbl)  [unwired: 2 in, 1 out]
                n843 = local write "Dielectric (d)"(w1891) -> ()
                n844 = local write "Threshold V"(w1892) -> ()
                n845 = local write "New Dielectric"(w1891) -> ()
                n846 = Decimate 1D Array(w1899) -> (w1900:cluster{dbl[], dbl[]}[])  [unwired: 1 out]
                n847 = Array To Cluster(array=w1900) -> (cluster=w1902:T5)
                n848 = local write "Table Control"(w1935) -> ()
                n849 = Unbundle(w1902) -> ("[0]"=w1901:cluster{dbl[], dbl[]})  [unwired: 8 out]
                n850 = Unbundle(w1901) -> (w1882:dbl[], w1881:dbl[])
                n851 = local write "XY Graph"(w1899) -> ()
                n852 = local write "Table Control 2"(w1934) -> ()
                n853 = local write "Mobility"(w1933) -> ()
                n854 = Array Subset(array=w1882, index=w1896, length=w1886) -> (w1898:dbl[])
                n855 = Array Subset(array=w1881, index=w1896, length=w1886) -> (w1897:dbl[])
                n856 = local write "Width"(w1890) -> ()
                n857 = local write "Length"(w1889) -> ()
                n858 = local write "Array 2"(w1897) -> ()
                n859 = Unbundle(w1872) -> ("Vt"=w1871:dbl, "STS"=w1870:dbl, "On/Off"=w1869:dbl)  [unwired: 4 out]
                n860 = local write "On/Off"(w1869) -> ()
                n861 = local write "Array"(w1898) -> ()
                n862 = local write "Slide"(w1896) -> ()
                n863 = local write "Index"(w1896) -> ()
                n864 = local write "STS recorded"(w1870) -> ()
                n865 = local write "Vt recorded"(w1871) -> ()
                n866 = Array Subset(array=w1874, index=w1880, length=w1879) -> (w1884:dbl[])
                n867 = Array Subset(array=w1873, index=w1880, length=w1879) -> (w1883:dbl[])
                n868 = local write "New Width"(w1890) -> ()
                n869 = local write "Data File"(w1887) -> ()
                n870 = local write "New Length"(w1889) -> ()
                n871 = local write "Array 8"(w1884) -> ()
                n872 = local write "Array 7"(w1883) -> ()
                n873 = call-poly <vilib>:"Read From Spreadsheet File.vi"("file path (dialog if empty)"=w1887) -> ("all rows"=w1922:string[][])  [unwired: 6 in, 4 out]
                n874 = local read "Image Folder"() -> (w1910:path)
                n875 = Array Size(array=w1922) -> (size(s)=w1921:i32[])
                n876 = List Folder(path=w1910) -> (filenames=w1915:string[])  [unwired: 3 in, 3 out]
                n877 = Index Array(array=w1921, index=w1920) -> (element=w1894:i32)
                n878 = Subtract(x=w1894, y=20) -> (x-y=w1893:i32)
                n879 = property on="Slide" class="Slide (strict)"("Scale.Maximum"=w1893) -> ()  [unwired: 2 in, 2 out]
                n880 = Array Subset(array=w1922, index (row)=w1920, index (col)=w1920, length (col)=3) -> (w1923:string[][])  [unwired: 1 in]
                n881 = Reshape Array(w1923, w1894) -> (w1903:string[])
                n882 = Search 1D Array(1D array=w1903, element="Mobility (cm^2/Vs):") -> (index of element=w1908:i32)  [unwired: 1 in]
                n883 = Search 1D Array(1D array=w1903, element="Index:") -> (index of element=w1917:i32)  [unwired: 1 in]
                n884 = Increment(x=w1917) -> (x+1=w1918:i32)
                n885 = Index Array(array=w1903, index=w1918) -> (element=w1913:string)
                n886 = while {
                  tunnel: w1915 -> [w1947]
                  tunnel: w1913 -> [w1945]
                  tunnel: [w1944] -> _
                  tunnel: [w1944] -> w1914
                  tunnel: w1894 -> [w1943]
                  i -> [w1944]
                  stop <- w1940 stop-if-true
                  n887 = Index Array(array=w1947, index=w1944) -> (element=w1948:string)
                  n888 = xnode "Match Regular Expression"("input string"=w1948, "regular expression"=w1945) -> ("whole match"=w1946:string)  [unwired: 4 in, 4 out]
                  n889 = Equal?(x=w1946, y=w1945) -> (x = y?=w1942:bool)
                  n890 = Equal?(x=w1943, y=w1944) -> (x = y?=w1941:bool)
                  n891 = Or(x=w1942, y=w1941) -> (x .or. y?=w1940:bool)
                }
                n892 = local write "Index 3"(w1913) -> ()
                n893 = Increment(x=w1908) -> (x+1=w1907:i32)
                n894 = local read "No Image"() -> (w1865:path)
                n895 = Index Array(array=w1903, index=w1907) -> (element=w1905:string)
                n896 = Fract/Exp String To Number(string=w1905) -> (number=w1904:dbl)  [unwired: 3 in, 1 out]
                n897 = local write "Recorded Mobility"(w1904) -> ()
                n898 = Path To String(path=w1910) -> (string=w1912:string)
                n899 = local read "Image Out"() -> (w1857:T2)
                n900 = Index Array(array=w1915, index=w1914) -> (element=w1867:string)
                n901 = Empty String/Path?(string/path=w1867) -> (empty?=w1868:bool)
                n902 = Concatenate Strings(w1912, "\\", w1867) -> (w1911:string)
                n903 = local write "Image Name"(w1867) -> ()
                n904 = String To Path(string=w1911) -> (path=w1866:path)
                n905 = Select(t=w1865, s=w1868, f=w1866) -> (s? t:f=w1859:path)
                n906 = local write "Image File"(w1859) -> ()
                n907 = call "IMAQ ReadFile"("File Path"=w1859, "Image"=w1857) -> ("Image Out"=w1858:T2)  [unwired: 5 in, 4 out]
                n908 = local write "Image Out 2"(w1858) -> ()
                n909 = local write "Image Out"(w1858) -> ()
                n910 = invoke on="Image Out" class="ImageControl" method="Clear ROI"() -> ()  [unwired: 3 in, 3 out]
              }
              frame #4 {
                n911 = local read "Image Folder"() -> (w2063:path)
                n912 = Build Path(base path=w2063, name or relative path="ROI") -> (appended path=w2065:path)
                n913 = local read "Index 3"() -> (w2064:string)
                n914 = Build Path(base path=w2065, name or relative path=w2064) -> (appended path=w2070:path)
                n915 = invoke on="Image Out" class="ImageControl" method="Clear ROI"() -> (error out=w2069:errorcluster)  [unwired: 3 in, 2 out]
                n916 = call <vilib>:"Check if File or Folder Exists.vi"("error in (no error)"=w2069, "path"=w2070) -> ("file or folder exists?"=w2067:bool, "dup path"=w2068:path)  [unwired: 7 in, 1 out]
                n917 = case shown="True" w2067 {
                  tunnel: w2068 -> [_ w2071]
                  frame False {
                  }
                  frame True {
                    n918 = Read from Text File(file (use dialog)=w2071) -> (text=w2075:string)  [unwired: 3 in, 3 out]
                    n919 = property on="Image Out" class="ImageControl"() -> ("ROI"=w2072:T7)  [unwired: 2 in, 2 out]
                    n920 = Unflatten From String(type=w2072, binary string=w2075) -> (value=w2073:T7, error out=w2074:errorcluster)  [unwired: 3 in, 1 out]
                    n921 = property on="Image Out" class="ImageControl"(error in=w2074, "ROI"=w2073) -> ()  [unwired: 1 in, 2 out]
                  }
                }
              }
              frame #5 {
                w2114 = "/"
                n922 = local read "Date Recorded"() -> (w2111:string)
                n923 = local read "Index 3"() -> (w2167:string)
                n924 = Match Pattern(string=w2111, regular expression=w2114) -> (before substring=w2120:string, after substring=w2113:string)  [unwired: 1 in, 2 out]
                n925 = String Length(string=w2120) -> (length=w2117:i32)
                n926 = Match Pattern(string=w2113, regular expression=w2114) -> (before substring=w2126:string, after substring=w2115:string)  [unwired: 1 in, 2 out]
                n927 = Equal?(x=w2117, y=2) -> (x = y?=w2119:bool)
                n928 = String Subset(string=w2167, length (rest)=1) -> (substring=w2087:string)  [unwired: 1 in]
                n929 = local write "Row"(w2087) -> ()
                n930 = String Length(string=w2126) -> (length=w2124:i32)
                n931 = Equal?(x=w2124, y=2) -> (x = y?=w2122:bool)
                n932 = String Subset(string=w2167, offset (0)=1, length (rest)=2) -> (substring=w2086:string)
                n933 = case shown="False" w2122 {
                  tunnel: w2126 -> [w2170 w2172]
                  tunnel: [w2169 w2172] -> w2125
                  frame False {
                    n934 = Concatenate Strings("0", w2170) -> (w2169:string)
                  }
                  frame True {
                  }
                }
                n935 = case shown="False" w2119 {
                  tunnel: w2120 -> [w2174 w2176]
                  tunnel: [w2173 w2176] -> w2121
                  frame False {
                    n936 = Concatenate Strings("0", w2174) -> (w2173:string)
                  }
                  frame True {
                  }
                }
                n937 = Build Array("DeviceID", "Fabricator", "Deposition", "Date", "Sample", "Row", "Column", "L (um)", "W (um)", "Material", "Treatment", "TC (mM)", "Solvent", "C (%)", "ST (C)", "Drops", "Wait (s)", "RT (F)", "RH (%)", "Ramp (s)", "RPM", "Accel (RPM/s)", "Time (s)", "Mobility", "On/Off", "Vt", "S.T.S") -> (w2084:string[])
                n938 = local write "Column"(w2086) -> ()
                n939 = local read "Wait Time (s):"() -> (w2077:dbl)
                n940 = local read "RPM:"() -> (w2081:dbl)
                n941 = local read "Index 3"() -> (w2127:string)
                n942 = local write "Transformer \nHeaders"(w2084) -> ()
                n943 = Number To Decimal String(number=w2077) -> (decimal integer string=w2078:string)  [unwired: 1 in]
                n944 = local read "Treatment Concentration (mM):"() -> (w2134:dbl)
                n945 = Number To Decimal String(number=w2081) -> (decimal integer string=w2080:string)  [unwired: 1 in]
                n946 = local read "Concentration Recorded"() -> (w2132:string)
                n947 = local read "# Drops:"() -> (w2092:dbl)
                n948 = local read "Relative Humidity (%):"() -> (w2137:dbl)
                n949 = local read "Solvent Recorded"() -> (w2133:string)
                n950 = local read "Solution Temp (C):"() -> (w2093:dbl)
                n951 = local read "Surface Treatment:"() -> (w2135:string)
                n952 = local read "Material Recorded"() -> (w2139:string)
                n953 = local read "Room Temp (F):"() -> (w2089:dbl)
                n954 = local read "Accel (RPM/s):"() -> (w2102:dbl)
                n955 = local read "New Mobility"() -> (w2100:dbl)
                n956 = local read "New Length"() -> (w2128:dbl)
                n957 = local read "New Width"() -> (w2129:dbl)
                n958 = local read "Sample #:"() -> (w2109:dbl)
                n959 = local read "New S.T.S."() -> (w2107:dbl)
                n960 = local read "Method Recorded"() -> (w2108:string)
                n961 = local read "Time (s):"() -> (w2097:dbl)
                n962 = Number To Decimal String(number=w2092) -> (decimal integer string=w2091:string)  [unwired: 1 in]
                n963 = local read "On/Off"() -> (w2103:dbl)
                n964 = local read "New Vt"() -> (w2105:dbl)
                n965 = local read "Date Recorded"() -> (w2112:string)
                n966 = local read "RPM:"() -> (w2096:dbl)
                n967 = local read "Fabricator:"() -> (w2088:string)
                n968 = Number To Decimal String(number=w2109) -> (decimal integer string=w2116:string)  [unwired: 1 in]
                n969 = call "DeviceID"("Sample"=w2116, "Year"=w2115, "Month"=w2121, "Day"=w2125, "Index"=w2127) -> ("Result"=w2110:string)  [unwired: 9 in, 1 out]
                n970 = Number To Decimal String(number=w2128) -> (decimal integer string=w2130:string)  [unwired: 1 in]
                n971 = Number To Decimal String(number=w2129) -> (decimal integer string=w2131:string)  [unwired: 1 in]
                n972 = Number To Decimal String(number=w2093) -> (decimal integer string=w2094:string)  [unwired: 1 in]
                n973 = Number To Decimal String(number=w2137) -> (decimal integer string=w2138:string)  [unwired: 1 in]
                n974 = Number To Decimal String(number=w2096) -> (decimal integer string=w2095:string)  [unwired: 1 in]
                n975 = Number To Fractional String(number=w2102, precision (6)=2) -> (F-format string=w2101:string)  [unwired: 2 in]
                n976 = Number To Decimal String(number=w2097) -> (decimal integer string=w2098:string)  [unwired: 1 in]
                n977 = Number To Fractional String(number=w2100) -> (F-format string=w2099:string)  [unwired: 3 in]
                n978 = Number To Fractional String(number=w2103) -> (F-format string=w2083:string)  [unwired: 3 in]
                n979 = Number To Fractional String(number=w2105) -> (F-format string=w2104:string)  [unwired: 3 in]
                n980 = Number To Fractional String(number=w2107) -> (F-format string=w2106:string)  [unwired: 3 in]
                n981 = Number To Decimal String(number=w2089) -> (decimal integer string=w2090:string)  [unwired: 1 in]
                n982 = Number To Decimal String(number=w2134) -> (decimal integer string=w2136:string)  [unwired: 1 in]
                n983 = Build Array(w2110, w2088, w2108, w2112, w2116, w2087, w2086, w2130, w2131, w2139, w2135, w2136, w2133, w2132, w2094, w2091, w2078, w2090, w2138, w2080, w2095, w2101, w2098, w2099, w2083, w2104, w2106) -> (w2085:string[])
                n984 = local write "Current \nRecord"(w2085) -> ()
              }
            }
            n985 = flat-sequence {
              tunnel: [w1734] -> w1721
              tunnel: w1721 -> [w1748]
              frame #0 {
                # "Makes Empty File for Transformer Data"
                n986 = local read "Data Folder"() -> (w1723:path)
                n987 = Build Path(base path=w1723, name or relative path="Stats") -> (appended path=w1725:path)
                n988 = call <vilib>:"Check if File or Folder Exists.vi"("path"=w1725) -> ("file or folder exists?"=w1726:bool, "dup path"=w1727:path)  [unwired: 8 in, 1 out]
                n989 = case shown="False" w1726 {
                  tunnel: [w1731 w1733] -> w1728
                  tunnel: w1727 -> [w1732 w1733]
                  frame False {
                    n990 = Create Folder(path (use dialog)=w1732) -> (created path=w1731:path)  [unwired: 2 in, 2 out]
                  }
                  frame True {
                  }
                }
                n991 = Build Path(base path=w1728, name or relative path="Tranformer Data.txt") -> (appended path=w1730:path)
                n992 = call-poly <vilib>:"Write To Spreadsheet File.vi"("append to file? (new file:F)"=TRUE, "file path (dialog if empty)"=w1730) -> ()  [unwired: 6 in, 1 out]
              }
              frame #1 {
                # "Adds Headers if they don't exist"
                n993 = Concatenate Strings("Stats\\", "Tranformer Data.txt") -> (w1741:string)
                n994 = local read "Data Folder"() -> (w1740:path)
                n995 = Build Path(base path=w1740, name or relative path=w1741) -> (appended path=w1734:path)
                n996 = call-poly <vilib>:"Read From Spreadsheet File.vi"("file path (dialog if empty)"=w1734) -> ("first row"=w1739:string[])  [unwired: 6 in, 4 out]
                n997 = Search 1D Array(1D array=w1739, element="DeviceID") -> (index of element=w1737:i32)  [unwired: 1 in]
                n998 = Equal?(x=w1737, y=0) -> (x = y?=w1735:bool)
                n999 = case shown="False" w1735 {
                  tunnel: w1734 -> [w1745 _]
                  frame False {
                    n1000 = local read "Transformer \nHeaders"() -> (w1744:string[])
                    n1001 = call-poly <vilib>:"Write To Spreadsheet File.vi"("1D data"=w1744, "file path (dialog if empty)"=w1745) -> ()  [unwired: 6 in, 1 out]
                  }
                  frame True {
                  }
                }
              }
              frame #2 {
                # "Adds current device if it doesn't exist"
                n1002 = local read "Current \nRecord"() -> (w1751:string[])
                n1003 = Index Array(array=w1751, index=0) -> (element=w1750:string)
                n1004 = Concatenate Strings("Stats\\", "Tranformer Data.txt") -> (w1754:string)
                n1005 = local read "Data Folder"() -> (w1753:path)
                n1006 = local write "Current Device ID"(w1750) -> ()
                n1007 = local read "Current Device ID"() -> (w1760:string)
                n1008 = Build Path(base path=w1753, name or relative path=w1754) -> (appended path=w1752:path)
                n1009 = call-poly <vilib>:"Read From Spreadsheet File.vi"("file path (dialog if empty)"=w1752) -> ("all rows"=w1747:string[][])  [unwired: 6 in, 4 out]
                n1010 = Index Array(array=w1747, index (col)=0) -> (element=w1758:string[])  [unwired: 1 in]
                n1011 = Search 1D Array(1D array=w1758, element=w1760) -> (index of element=w1746:i32)  [unwired: 1 in]
                n1012 = Equal?(x=w1746, y=-1) -> (x = y?=w1749:bool)
                n1013 = case shown="False" w1749 {
                  tunnel: w1748 -> [w1762 w1775]
                  tunnel: w1746 -> [w1767 _]
                  tunnel: w1747 -> [w1768 _]
                  frame False {
                    n1014 = local read "Current \nRecord"() -> (w1766:string[])
                    n1015 = Replace Array Subset(array=w1768, new element=w1766, index (row)=w1767) -> (w1763:string[][])  [unwired: 1 in]
                    n1016 = flat-sequence {
                      tunnel: [w1769] -> _
                      tunnel: [w1770] -> _
                      tunnel: [w1770] -> w1765
                      tunnel: [w1769] -> w1764
                      tunnel: w1763 -> [w1770]
                      tunnel: w1762 -> [w1769]
                      tunnel: w1765 -> [w1772]
                      tunnel: w1764 -> [w1771]
                      frame #0 {
                        n1017 = Delete(path (use dialog)=w1769) -> ()  [unwired: 4 in, 3 out]
                      }
                      frame #1 {
                        n1018 = call-poly <vilib>:"Write To Spreadsheet File.vi"("append to file? (new file:F)"=TRUE, "2D data"=w1772, "file path (dialog if empty)"=w1771) -> ()  [unwired: 5 in, 1 out]
                      }
                    }
                  }
                  frame True {
                    n1019 = local read "Current \nRecord"() -> (w1774:string[])
                    n1020 = call-poly <vilib>:"Write To Spreadsheet File.vi"("append to file? (new file:F)"=TRUE, "1D data"=w1774, "file path (dialog if empty)"=w1775) -> ()  [unwired: 5 in, 1 out]
                  }
                }
              }
            }
          }
          event "Export": Mouse Down {
            n1021 = event-data() -> ()  [unwired: 1 in, 7 out]
            n1022 = call "OA_ConnectToOrigin.vi"() -> ("error out"=w2198:errorcluster, "Origin.IOApplication"=w2199:refnum<k7>)  [unwired: 8 in]
            n1023 = local read "Data Folder"() -> (w2177:path)
            n1024 = local read "Project"() -> (w2197:path)
            n1025 = call "OA_Load.vi"("error in (no error)"=w2198, "Path"=w2197, "Origin.IOApplication"=w2199) -> ("error out"=w2190:errorcluster, "Origin.IOApplication"=w2191:refnum<k7>)  [unwired: 1 out]
            n1026 = call "OAExecute.vi"("script"="document -m 3;", "Error IO"=w2190, "Origin.IOApplication"=w2191) -> ("Error IO Out"=w2188:errorcluster, "Origin.IOApplication"=w2189:refnum<k7>)  [unwired: 1 in, 1 out]
            n1027 = Build Path(base path=w2177, name or relative path="Stats") -> (appended path=w2178:path)
            n1028 = flat-sequence {
              tunnel: w2177 -> [w2219]
              tunnel: w2196 -> [w2218]
              tunnel: [w2208] -> w2201
              tunnel: [w2209] -> w2200
              tunnel: w2189 -> [w2213]
              tunnel: w2188 -> [w2212]
              tunnel: w2177 -> [w2235]
              tunnel: w2196 -> [w2234]
              tunnel: w2201 -> [w2230]
              tunnel: w2200 -> [w2231]
              tunnel: [w2225] -> w2195
              tunnel: [w2224] -> w2194
              tunnel: w2177 -> [w2246]
              tunnel: w2196 -> [w2245]
              tunnel: w2195 -> [w2241]
              tunnel: w2194 -> [w2240]
              tunnel: [w2239] -> w2193
              tunnel: [w2238] -> w2192
              tunnel: w2177 -> [w2261]
              tunnel: w2196 -> [w2260]
              tunnel: w2193 -> [w2255]
              tunnel: w2192 -> [w2254]
              tunnel: [w2252] -> w2186
              tunnel: [w2251] -> w2185
              frame #0 {
                n1029 = call "Param_Analysis.vi"("error in (no error)"=w2212, "Folder 2"=w2219, "Parameter String"="Mobility (cm^2/Vs):", "Parameter Name"="Mobility", "Folder"=w2218) -> ("error out"=w2215:errorcluster, "Array 4"=w2205:string[], "Array 3"=w2214:string[][])  [unwired: 3 in, 1 out]
                n1030 = call "Origin_Export.vi"("String 3"="[MobHistTab]Sheet1", "error in (no error)"=w2215, "Array"=w2214, "String 2"="[MOBvsLTable]Mobilities", "String"="pe_cd \"Mobility Chart\";", "Origin.IOApplication"=w2213, "Array 2"=w2205) -> ("reference out"=w2211:refnum<k7>, "error out"=w2210:errorcluster)  [unwired: 2 in, 1 out]
                n1031 = call "OAExecute.vi"("script"="window -a MOBvsLTable;\nwindow -s TV;", "Error IO"=w2210, "Origin.IOApplication"=w2211) -> ("Error IO Out"=w2208:errorcluster, "Origin.IOApplication"=w2209:refnum<k7>)  [unwired: 1 in, 1 out]
              }
              frame #1 {
                n1032 = call "Param_Analysis.vi"("error in (no error)"=w2230, "Folder 2"=w2235, "Parameter String"="On/Off Current:", "Parameter Name"="On_Off_Current", "Folder"=w2234) -> ("error out"=w2229:errorcluster, "Array 4"=w2223:string[], "Array 3"=w2226:string[][])  [unwired: 3 in, 1 out]
                n1033 = call "Origin_Export.vi"("String 3"="[OnOffHistTab]Sheet1", "error in (no error)"=w2229, "Array"=w2226, "String 2"="[OnOffTable]On/Off Ratios", "String"="pe_cd \"OnOff vs L\";", "Origin.IOApplication"=w2231, "Array 2"=w2223) -> ("reference out"=w2225:refnum<k7>, "error out"=w2224:errorcluster)  [unwired: 2 in, 1 out]
              }
              frame #2 {
                n1034 = call "Param_Analysis.vi"("Folder 2"=w2246, "Parameter String"="S.T.S. (V/decade):", "Parameter Name"="STS", "Folder"=w2245) -> ("Array 4"=w2237:string[], "Array 3"=w2242:string[][])  [unwired: 4 in, 2 out]
                n1035 = call "Origin_Export.vi"("String 3"="[SHistTab]Sheet1", "error in (no error)"=w2240, "Array"=w2242, "String 2"="[STable]Threshold Swing", "String"="pe_cd \"Threshold Swing vs L\";", "Origin.IOApplication"=w2241, "Array 2"=w2237) -> ("reference out"=w2238:refnum<k7>, "error out"=w2239:errorcluster)  [unwired: 2 in, 1 out]
              }
              frame #3 {
                n1036 = call "Param_Analysis.vi"("Folder 2"=w2261, "Parameter String"="Threshold V (V):", "Parameter Name"="Threshold_V", "Folder"=w2260) -> ("Array 4"=w2250:string[], "Array 3"=w2253:string[][])  [unwired: 4 in, 2 out]
                n1037 = call "Origin_Export.vi"("String 3"="[VtHistTab]Sheet1", "error in (no error)"=w2255, "Array"=w2253, "String 2"="[VtTable]Threshold Voltages", "String"="pe_cd \"Threshold Voltage vs L\";", "Origin.IOApplication"=w2254, "Array 2"=w2250) -> ("reference out"=w2252:refnum<k7>, "error out"=w2251:errorcluster)  [unwired: 2 in, 1 out]
              }
            }
            n1038 = call <vilib>:"Check if File or Folder Exists.vi"("path"=w2178) -> ("file or folder exists?"=w2203:bool, "dup path"=w2202:path)  [unwired: 8 in, 1 out]
            n1039 = case shown="False" w2203 {
              tunnel: w2202 -> [w2263 w2264]
              tunnel: [w2262 w2264] -> w2196
              frame False {
                n1040 = Create Folder(path (use dialog)=w2263) -> (created path=w2262:path)  [unwired: 2 in, 2 out]
              }
              frame True {
              }
            }
            n1041 = call "File Dialog"("start path"=w2178) -> ("selected path"=w2181:path)  [unwired: 11 in, 3 out]
            n1042 = Path To String(path=w2181) -> (string=w2180:string)
            n1043 = call "OAExecute.vi"("script"="pe_cd /;\npe_cd \"Mobility Chart\"; ", "Error IO"=w2185, "Origin.IOApplication"=w2186) -> ("Error IO Out"=w2182:errorcluster, "Origin.IOApplication"=w2183:refnum<k7>)  [unwired: 1 in, 1 out]
            n1044 = call "OASaveProject.vi"("path"=w2180, "Error IO"=w2182, "Origin.IOApplication"=w2183) -> ()  [unwired: 3 out]
          }
          event "Blank Button": Mouse Down {
            n1045 = event-data() -> ()  [unwired: 1 in, 7 out]
            n1046 = local read "Data File"() -> (w2272:path)
            n1047 = Strip Path(path=w2272) -> (stripped path=w2268:path, name=w2270:string)
            n1048 = Path To String(path=w2268) -> (string=w2267:string)
            n1049 = Concatenate Strings(w2267, "\\", "X_", w2270) -> (w2266:string)
            n1050 = String To Path(string=w2266) -> (path=w2265:path)
            n1051 = Move(source path=w2272, 10:w2265) -> ()  [unwired: 3 in, 3 out]
            n1052 = local write "Data File"(w2265) -> ()
          }
          event "Cancel Button": Mouse Down {
            (unwired) 6
            n1053 = event-data() -> ()  [unwired: 1 in, 7 out]
            n1054 = call "Simulate_Keyboard.vi"("Action"=2, "Virtual Key"=162) -> ()  [unwired: 7 in, 1 out]
          }
        }
        n1055 = property on="Image Out" class="ImageControl"() -> ("ROI"=w366:T7)  [unwired: 2 in, 2 out]
        n1056 = local read "Image Out"() -> (w395:T2)
        n1057 = property on="Image Out" class="ImageControl"() -> ("ZoomSingle"=w409:cluster{"X":sgl, "Y":sgl})  [unwired: 2 in, 2 out]
        n1058 = property on="Image Out" class="ImageControl"() -> ("Bounds"=w410:T8)  [unwired: 2 in, 2 out]
        n1059 = Unbundle By Name(w366) -> ("Contours"=w440:T9)
        n1060 = call <vilib>:"Intialize Keyboard.vi"() -> ("device ID"=w421:refnum<k1>)  [unwired: 10 in, 1 out]
        n1061 = property on="Image Out" class="ImageControl"() -> ("Image Center Position"=w416:cluster{"X":u32, "Y":u32})  [unwired: 2 in, 2 out]
        n1062 = call "IMAQ Clear Overlay"("Image"=w395) -> ("Image Out"=w394:T2)  [unwired: 9 in, 1 out]
        n1063 = call-poly <vilib>:"Acquire Input Data.vi"("device ID"=w421) -> ("keys pressed"=w420:T10)  [unwired: 16 in, 2 out]
        n1064 = Initialize Array(0) -> (w438:i32[])  [unwired: 1 in]
        n1065 = local read "Magnification"() -> (w429:u16)
        n1066 = Unbundle(w410) -> ("Width"=w407:u32, "Height"=w406:u32)
        n1067 = Array Size(array=w440) -> (size(s)=w439:i32)
        n1068 = Unbundle(w409) -> ("X"=w384:sgl, "Y"=w408:sgl)
        n1069 = event shown="[2] \" Image Folder\": Value Change" {
          selector: _ -> [_ _ _ _ _ _ _]
          dyn-events: _ -> [_ _ _ _ _ _ _]
          timeout: 10 -> [_ _ _ _ _ _ _]
          event "Remove Button": Mouse Down {
            w446 = 0
            n1070 = property on="Image Out" class="ImageControl"() -> ("ROI"=w444:T7)  [unwired: 2 in, 2 out]
            n1071 = event-data() -> ()  [unwired: 1 in, 7 out]
            n1072 = Unbundle(w444) -> ("Global Rectangle"=w447:i32[], "Contours"=w449:T9)
            n1073 = Reverse 1D Array(array=w447) -> (reversed array=w448:i32[])
            n1074 = Reverse 1D Array(array=w449) -> (reversed array=w450:T9)
            n1075 = Delete From Array(array=w448, index=w446) -> (array with subset deleted=w451:i32[])  [unwired: 1 in, 1 out]
            n1076 = Delete From Array(array=w450, index=w446) -> (array with subset deleted=w452:T9)  [unwired: 1 in, 1 out]
            n1077 = Reverse 1D Array(array=w451) -> (reversed array=w453:i32[])
            n1078 = Reverse 1D Array(array=w452) -> (reversed array=w454:T9)
            n1079 = Bundle(w453, w454) -> (w445:T11)  [unwired: 1 in]
            n1080 = local write "ROI Descriptor out"(w444) -> ()
            n1081 = local write "ROI Descriptor"(w445) -> ()
            n1082 = property on="Image Out" class="ImageControl"("ROI"=w445) -> ()  [unwired: 2 in, 2 out]
          }
          event "Undo Button": Mouse Down {
            n1083 = event-data() -> ()  [unwired: 1 in, 7 out]
            n1084 = invoke on="Image Out" class="ImageControl" method="Clear ROI"() -> ()  [unwired: 3 in, 3 out]
          }
          event "Image Folder": Value Change {
            n1085 = event-data() -> ()  [unwired: 1 in, 5 out]
            n1086 = local read "Image File"() -> (w456:path)
            n1087 = call "Vision Acquisition"("Image Path"=w456) -> ("Image Out"=w455:T2)  [unwired: 25 in, 1 out]
            n1088 = local write "Image Out 2"(w455) -> ()
            n1089 = local write "Image Out"(w455) -> ()
            n1090 = invoke on="Image Out" class="ImageControl" method="Clear ROI"() -> ()  [unwired: 3 in, 3 out]
          }
          event "Zoom": Value Change {
            n1091 = event-data() -> ()  [unwired: 1 in, 5 out]
            n1092 = local read "Zoom"() -> (w457:i16)
            n1093 = Bundle("Zoom"=w457, "Zoom"=w457) -> (w458:cluster{"Zoom":i16, "Zoom":i16})  [unwired: 1 in]
            n1094 = property on="Image Out" class="ImageControl"("ZoomInteger"=w458) -> ()  [unwired: 2 in, 2 out]
          }
          event Timeout {
            n1095 = event-data() -> ()  [unwired: 1 in, 2 out]
          }
          event "Image Out": Mouse Enter {
            (unwired) 6
            n1096 = event-data() -> ()  [unwired: 1 in, 3 out]
            n1097 = call "Simulate_Keyboard.vi"("Action"=0, "Virtual Key"=162) -> ()  [unwired: 7 in, 1 out]
          }
          event "Image Out": Mouse Leave {
            n1098 = event-data() -> ()  [unwired: 1 in, 3 out]
            n1099 = flat-sequence {
              frame #0 {
                n1100 = Wait (ms)(milliseconds to wait=10) -> ()  [unwired: 1 out]
              }
              frame #1 {
                (unwired) 6
                n1101 = call "Simulate_Keyboard.vi"("Action"=2, "Virtual Key"=162) -> ()  [unwired: 7 in, 1 out]
              }
            }
          }
        }
        n1102 = Build Array(0.505025, 0.252522, 0.127742, 0.050345, 0.031129) -> (w430:dbl[])
        n1103 = Index Array(array=w420) -> (element=w424:T12)  [unwired: 1 in]
        n1104 = Divide(x=w407, y=w384) -> (x/y=w397:sgl)
        n1105 = Multiply(x=w397, y=0.5) -> (x*y=w403:dbl)
        n1106 = Divide(x=w406, y=w408) -> (x/y=w396:sgl)
        n1107 = Multiply(x=w396, y=0.5) -> (x*y=w402:dbl)
        n1108 = Array Subset(array=w430, index=w429, length=1) -> (w427:dbl[])
        n1109 = property on="Image Out" class="ImageControl"() -> ("ZoomInteger"=w419:cluster{"X":i32, "Y":i32})  [unwired: 2 in, 2 out]
        n1110 = Unbundle(w416) -> ("X"=w398:u32, "Y"=w399:u32)
        n1111 = Subtract(x=w399, y=w402) -> (x-y=w400:dbl)
        n1112 = Subtract(x=w398, y=w403) -> (x-y=w401:dbl)
        n1113 = Add(x=w401, y=w397) -> (x+y=w415:dbl)
        n1114 = Add(x=w400, y=w396) -> (x+y=w414:dbl)
        n1115 = To Double Precision Float(number=w427) -> (double precision float=w426:dbl[])
        n1116 = local write "ROI Descriptor"(w366) -> ()
        n1117 = Reciprocal(x=w384) -> (1/x=w383:sgl)
        n1118 = Unbundle(w419) -> ("X"=w418:i32)  [unwired: 1 out]
        n1119 = Multiply(x=w383, y=10) -> (x*y=w385:sgl)
        n1120 = case shown="\"EQUALS\"" w424 {
          tunnel: w398 -> [w465 w471 w475 w477 w481 w483 w485 w487 w489 w491 w493 w495 w497 w499 w501 w503 w505 w507 w509 w511 w513 w515 w517 w519 w521 w523 w525 w527 w529 w531 w533 w535 w537 w539 w541 w543 w545 w547 w549 w551 w553 w555 w557 w559 w561 w563 w565 w567 w569 w571 w573 w575 w577 w579 w581 w583 w585 w587 w589 w591 w593 w595 w597 w599 w601 w603 w605 w607 w609 w611 w613 w615 w617 w619 w621 w623 w625 w627 w629 w631 w633 w635 w637 w639 w641 w643 w645 w647 w649 w651 w653 w655 w657 w659 w661 w663 w665 w667 w669 w671 w673 w675 w677 w679 w681]
          tunnel: [w465 w470 w474 w477 w481 w483 w485 w487 w489 w491 w493 w495 w497 w499 w501 w503 w505 w507 w509 w511 w513 w515 w517 w519 w521 w523 w525 w527 w529 w531 w533 w535 w537 w539 w541 w543 w545 w547 w549 w551 w553 w555 w557 w559 w561 w563 w565 w567 w569 w571 w573 w575 w577 w579 w581 w583 w585 w587 w589 w591 w593 w595 w597 w599 w601 w603 w605 w607 w609 w611 w613 w615 w617 w619 w621 w623 w625 w627 w629 w631 w633 w635 w637 w639 w641 w643 w645 w647 w649 w651 w653 w655 w657 w659 w661 w663 w665 w667 w669 w671 w673 w675 w677 w679 w681] -> w423
          tunnel: w399 -> [w467 w469 w473 w479 w480 w482 w484 w486 w488 w490 w492 w494 w496 w498 w500 w502 w504 w506 w508 w510 w512 w514 w516 w518 w520 w522 w524 w526 w528 w530 w532 w534 w536 w538 w540 w542 w544 w546 w548 w550 w552 w554 w556 w558 w560 w562 w564 w566 w568 w570 w572 w574 w576 w578 w580 w582 w584 w586 w588 w590 w592 w594 w596 w598 w600 w602 w604 w606 w608 w610 w612 w614 w616 w618 w620 w622 w624 w626 w628 w630 w632 w634 w636 w638 w640 w642 w644 w646 w648 w650 w652 w654 w656 w658 w660 w662 w664 w666 w668 w670 w672 w674 w676 w678 w680]
          tunnel: [w466 w469 w473 w478 w480 w482 w484 w486 w488 w490 w492 w494 w496 w498 w500 w502 w504 w506 w508 w510 w512 w514 w516 w518 w520 w522 w524 w526 w528 w530 w532 w534 w536 w538 w540 w542 w544 w546 w548 w550 w552 w554 w556 w558 w560 w562 w564 w566 w568 w570 w572 w574 w576 w578 w580 w582 w584 w586 w588 w590 w592 w594 w596 w598 w600 w602 w604 w606 w608 w610 w612 w614 w616 w618 w620 w622 w624 w626 w628 w630 w632 w634 w636 w638 w640 w642 w644 w646 w648 w650 w652 w654 w656 w658 w660 w662 w664 w666 w668 w670 w672 w674 w676 w678 w680] -> w422
          tunnel: w385 -> [w464 w468 w472 w476 _ _ _ _ _ _ _ _ _ _ _ _ _ _ _ _ _ _ _ _ _ _ _ _ _ _ _ _ _ _ _ _ _ _ _ _ _ _ _ _ _ _ _ _ _ _ _ _ _ _ _ _ _ _ _ _ _ _ _ _ _ _ _ _ _ _ _ _ _ _ _ _ _ _ _ _ _ _ _ _ _ _ _ _ _ _ _ _ _ _ _ _ _ _ _ _ _ _ _ _ _]
          frame "DOWN" {
            n1121 = Add(x=w467, y=w464) -> (x+y=w466:sgl)
          }
          frame "LEFT" {
            n1122 = Subtract(x=w471, y=w468) -> (x-y=w470:sgl)
          }
          frame "RIGHT" {
            n1123 = Add(x=w475, y=w472) -> (x+y=w474:sgl)
          }
          frame "UP" {
            n1124 = Subtract(x=w479, y=w476) -> (x-y=w478:sgl)
          }
          frame "ENTER (num pad)" {
          }
          frame "' (quote)" {
          }
          frame "END" {
          }
          frame "EQUALS" {
          }
          frame "ESCAPE" {
          }
          frame "GRAVE (`)" {
          }
          frame "HOME" {
          }
          frame "INSERT" {
          }
          frame "LBRACKET" {
          }
          frame "LCONTROL" {
          }
          frame "L ALT" {
          }
          frame "LSHIFT" {
          }
          frame "LWIN" {
          }
          frame "MINUS" {
          }
          frame "MULTIPLY" {
          }
          frame "NEXT" {
          }
          frame "NUMLOCK" {
          }
          frame "NUMPAD_0" {
          }
          frame "NUMPAD_1" {
          }
          frame "NUMPAD_2" {
          }
          frame "NUMPAD_3" {
          }
          frame "NUMPAD_4" {
          }
          frame "NUMPAD_5" {
          }
          frame "NUMPAD_6" {
          }
          frame "NUMPAD_7" {
          }
          frame "NUMPAD_8" {
          }
          frame "NUMPAD_9" {
          }
          frame "PAUSE" {
          }
          frame "PERIOD" {
          }
          frame "PRIOR (PG UP)" {
          }
          frame "RBRACKET" {
          }
          frame "RCONTROL" {
          }
          frame "RETURN" {
          }
          frame "R ALT" {
          }
          frame "RSHIFT" {
          }
          frame "RWIN" {
          }
          frame "SCROLL" {
          }
          frame "SEMICOLON" {
          }
          frame "SLASH" {
          }
          frame "SPACE" {
          }
          frame "SUBTRACT" {
          }
          frame "TAB" {
          }
          frame "DIVIDE" {
          }
          frame "DELETE" {
          }
          frame "DECIMAL" {
          }
          frame "COMMA" {
          }
          frame "CAPITAL" {
          }
          frame "BACKSLASH" {
          }
          frame "BACK" {
          }
          frame "ADD" {
          }
          frame "F15" {
          }
          frame "F14" {
          }
          frame "F13" {
          }
          frame "F12" {
          }
          frame "F11" {
          }
          frame "F10" {
          }
          frame "F9" {
          }
          frame "F8" {
          }
          frame "F7" {
          }
          frame "F6" {
          }
          frame "F5" {
          }
          frame "F4" {
          }
          frame "F3" {
          }
          frame "F2" {
          }
          frame "F1" {
          }
          frame "Z" {
          }
          frame "Y" {
          }
          frame "X" {
          }
          frame "W" {
          }
          frame "V" {
          }
          frame "U" {
          }
          frame "T" {
          }
          frame "S" {
          }
          frame "R" {
          }
          frame "Q" {
          }
          frame "P" {
          }
          frame "O" {
          }
          frame "N" {
          }
          frame "M" {
          }
          frame "L" {
          }
          frame "K" {
          }
          frame "J" {
          }
          frame "I" {
          }
          frame "H" {
          }
          frame "G" {
          }
          frame "F" {
          }
          frame "E" {
          }
          frame "D" {
          }
          frame "C" {
          }
          frame "B" {
          }
          frame "A" {
          }
          frame "9" {
          }
          frame "8" {
          }
          frame "7" {
          }
          frame "6" {
          }
          frame "5" {
          }
          frame "4" {
          }
          frame "3" {
          }
          frame "2" {
          }
          frame "1" {
          }
          frame "0" {
          }
        }
        n1125 = Bundle(w401, w400, w415, w414, 0.0) -> (w413:cluster{dbl, dbl, dbl, dbl, dbl})  [unwired: 1 in]
        n1126 = Bundle("X"=w423, "Y"=w422) -> (w417:cluster{"X":sgl, "Y":sgl})  [unwired: 1 in]
        n1127 = Divide(x=20, y=w384) -> (x/y=w387:sgl)
        n1128 = local write "Zoom"(w418) -> ()
        n1129 = property on="Image Out" class="ImageControl"("Image Center Position"=w417) -> ()  [unwired: 2 in, 2 out]
        n1130 = call "IMAQ Convert Rectangle to ROI (Polygon)"("Rectangle"=w413) -> ("ROI Descriptor"=w411:T3)  [unwired: 7 in, 2 out]
        n1131 = Bundle("Application Font", w387, w391, w391, w391, w391, w391, TRUE, w389) -> (w393:T13)  [unwired: 1 in]
        n1132 = property on="Image Out 2" class="ImageControl"("ROI"=w411) -> ()  [unwired: 2 in, 2 out]
        n1133 = Bundle(w389, w393, w389, w389) -> (w392:T14)  [unwired: 1 in]
        n1134 = for {
          N: w439 -> [_]
          shift-right: [w704] -> _
          shift-left: w440 -> [w704]
          shift-right: [w702] -> w425
          shift-left: w438 -> [w701]
          tunnel: w426 -> [w700]
          shift-right: [w697] -> _
          shift-left: w394 -> [w699]
          tunnel: w392 -> [w692]
          i -> [w696]
          n1135 = Index Array(array=w704, index=w696) -> (element=w713:T15)
          n1136 = Unbundle(w713) -> ("Points"=w712:i32[])  [unwired: 2 out]
          n1137 = Array To Cluster(array=w712) -> (cluster=w711:T16)
          n1138 = Unbundle(w711) -> ("Points[0]"=w691:i32, "Points[1]"=w688:i32, "Points[2]"=w703:i32, "Points[3]"=w709:i32)  [unwired: 5 out]
          n1139 = Add(x=w691, y=10) -> (x+y=w689:i32)
          n1140 = Subtract(x=w688, y=w709) -> (x-y=w708:i32)
          n1141 = Subtract(x=w691, y=w703) -> (x-y=w710:i32)
          n1142 = Square(x=w708) -> (x^2=w706:i32)
          n1143 = Square(x=w710) -> (x^2=w707:i32)
          n1144 = Add(x=w707, y=w706) -> (x+y=w705:i32)
          n1145 = Square Root(x=w705) -> (sqrt(x)=w682:dbl)
          n1146 = Multiply(x=w682, y=0.5) -> (x*y=w685:dbl)
          n1147 = Add(x=w685, y=w688) -> (x+y=w687:dbl)
          n1148 = Bundle(w689, w687) -> (w698:cluster{i32, dbl})  [unwired: 1 in]
          n1149 = Multiply(x=w682, y=w700) -> (x*y=w695:dbl[])
          n1150 = Index Array(array=w695) -> (element=w694:dbl)  [unwired: 1 in]
          n1151 = Number To Fractional String(number=w694) -> (F-format string=w693:string)  [unwired: 3 in]
          n1152 = call "IMAQ Overlay Text"("BG Color (Transparent)"=u32 0, "Text Color (black)"=u32 16448250, "Font, Size & Style"=w692, "String"=w693, "Origin"=w698, "Image"=w699) -> ("Image Out"=w697:T2)  [unwired: 4 in, 1 out]
          n1153 = Build Array (concatenate)(w701, w695) -> (w702:dbl[])
          n1154 = local write "Numeric 3"(w682) -> ()
        }
        n1155 = Add Array Elements(numeric array=w425) -> (sum=w436:dbl)
        n1156 = local write "Distances"(w425) -> ()
        n1157 = local write "Total Width"(w436) -> ()
        n1158 = local read "Array 8"() -> (w371:dbl[])
        n1159 = local read "Array 7"() -> (w372:dbl[])
        n1160 = local read "Width"() -> (w367:dbl)
        n1161 = local read "New Dielectric"() -> (w379:dbl)
        n1162 = local read "Array 2"() -> (w375:dbl[])
        n1163 = local read "Manual"() -> (w365:bool)
        n1164 = local read "New Length"() -> (w377:dbl)
        n1165 = local read "Array"() -> (w376:dbl[])
        n1166 = call "sts_calc_subvi.vi"("Array 2"=w371, "Array"=w372) -> ("STS"=w373:dbl)  [unwired: 9 in]
        n1167 = local read "New Width"() -> (w380:dbl)
        n1168 = local write "New S.T.S."(w373) -> ()
        n1169 = call "mob_calc_subvi.vi"("Width"=w380, "Length"=w377, "Dielectric (d)"=w379, "Array 2"=w375, "Array"=w376) -> ("Vt"=w374:dbl, "Mobility"=w378:dbl)  [unwired: 5 in]
        n1170 = Not(x=w365) -> (.not. x?=w363:bool)
        n1171 = local write "New Vt"(w374) -> ()
        n1172 = local write "New Mobility"(w378) -> ()
        n1173 = local read "Total Width"() -> (w369:dbl)
        n1174 = Equal To 0?(x=w369) -> (x = 0?=w364:bool)
        n1175 = And(x=w364, y=w363) -> (x .and. y?=w362:bool)
        n1176 = case shown="True" w362 {
          tunnel: w367 -> [_ w442]
          frame False {
          }
          frame True {
            n1177 = local write "New Width"(w442) -> ()
          }
        }
        n1178 = Or(x=w364, y=w365) -> (x .or. y?=w368:bool)
        n1179 = case shown="False" w368 {
          tunnel: w369 -> [w443 _]
          frame False {
            n1180 = local write "New Width"(w443) -> ()
          }
          frame True {
          }
        }
      }
    }
  }
  n1181 = disable-structure shown="Disabled" {
    frame Disabled {
      n1182 = local read "Data Folder"() -> ()  [unwired: 1 out]
      n1183 = local read "Data Folder"() -> ()  [unwired: 1 out]
      n1184 = local read "Data Folder"() -> ()  [unwired: 1 out]
    }
    frame Enabled {
    }
  }
